vi "WS1050_Bench_Full Step_Hex_Characterization.vi"(4 "Send":bool, 5 "CLICK DOWN TO QUIT":bool=TRUE) -> (0 "EXE SEQ":bool, 1 "POWER ON":bool, 2 "CHARGE \nPUMP ON":bool, 3 "POWER OFF":bool)   [LabVIEW 2012]
panel:
  out "Con_HEX":string
  in  "Cmd Full":string[](array[string])=["01", "02", "03", "04", "05", "06", "07", "08", "09", "0A", "0B", "0C", "0D", "0E", "0F", "10", "11", "12", "13", "14", "15", "16", "17", "18", "19", "1A", "1B", "1C", "1D", "1E", "1F", "20", "21", "22", "23", "24", "25", "26", "27", "28", "29", "2A", "2B", "2C", "2D", "2E", "2F", "30", "31", "32", "33", "34", "35", "36", "37", "38", "39", "3A", "3B", "3A", "39", "38", "37", "36", "35", "34", "33", "32", "31", "30", "2F", "2E", "2D", "2C", "2B", "2A", "29", "28", "27", "26", "25", "24", "23", "22", "21", "20", "1F", "1E", "1D", "1C", "1B", "1A", "19", "18", "17", "16", "15", "14", "13", "12", "11", "10", "0F", "0E", "0D", "0C", "0B", "0A", "09", "08", "07", "06", "05", "04", "03", "02", "01", "00"]
  in  "Driver Name Full":string[](array[string])=["S0F1_UP", "S0F2_UP", "S0F12_UP", "S1_UP", "S1F1_UP", "S1F2_UP", "S1F12_UP", "S2_UP", "S2F1_UP", "S2F2_UP", "S2F12_UP", "S3_UP", "S3F1_UP", "S3F2_UP", "S3F12_UP", "S4_UP", "S4F1_UP", "S4F2_UP", "S4F12_UP", "S5_UP", "S5F1_UP", "S5F2_UP", "S5F12_UP", "S6_UP", "S6F1_UP", "S6F2_UP", "S6F12_UP", "S7_UP", "S7F1_UP", "S7F2_UP", "S7F12_UP", "S8_UP", "S8F1_UP", "S8F2_UP", "S8F12_UP", "S9_UP", "S9F1_UP", "S9F2_UP", "S9F12_UP", "S10_UP", "S10F1_UP", "S10F2_UP", "S10F12_UP", "S11_UP", "S11F1_UP", "S11F2_UP", "S11F12_UP", "S12_UP", "S12F1_UP", "S12F2_UP", "S12F12_UP", "S13_UP", "S13F1_UP", "S13F2_UP", "S13F12_UP", "S14_UP", "S14F1_UP", "S14F2_UP", "S14F12_UP", "S14F2_DN", "S14F1_DN", "S14_DN", "S13F12_DN", "S13F2_DN", "S13F1_DN", "S13_DN", "S12F12_DN", "S12F2_DN", "S12F1_DN", "S12_DN", "S11F12_DN", "S11F2_DN", "S11F1_DN", "S11_DN", "S10F12_DN", "S10F2_DN", "S10F1_DN", "S10_DN", "S9F12_DN", "S9F2_DN", "S9F1_DN", "S9_DN", "S8F12_DN", "S8F2_DN", "S8F1_DN", "S8_DN", "S7F12_DN", "S7F2_DN", "S7F1_DN", "S7_DN", "S6F12_DN", "S6F2_DN", "S6F1_DN", "S6_DN", "S5F12_DN", "S5F2_DN", "S5F1_DN", "S5_DN", "S4F12_DN", "S4F2_DN", "S4F1_DN", "S4_DN", "S3F12_DN", "S3F2_DN", "S3F1_DN", "S3_DN", "S2F12_DN", "S2F2_DN", "S2F1_DN", "S2_DN", "S1F12_DN", "S1F2_DN", "S1F1_DN", "S1_DN", "S0F12_DN", "S0F2_DN", "S0F1_DN", "ALL_OFF"]
  in  "Reg1_Bit Cntrl 2":string[](array[string])=["01", "02", "04", "08", "10", "20", "40", "80", "03", "06", "0C", "D8", "33", "66", "CC", "07", "0E", "1C", "38", "70", "E0", "0F", "1E", "3C", "78", "F0", "1F", "3E", "7C", "F8", "3F", "7E", "FC", "7F", "FE", "FD", "FB", "F7", "EF", "DF", "BF", "7F", "FC", "F9", "F3", "E7", "CF", "9F", "3F", "F8", "F1", "E3", "C7", "8F", "1F", "F0", "E1", "C3", "87", "0F", "E0", "C1", "83", "07", "C0", "81", "03", "AA", "55", "00"]
  out "CMin C3(pF)":dbl=-3.580591796875
  out "Delta_C3(pF)":dbl=11.179992796875
  out "CMin C2(pF)":dbl=-3.6213935546875
  out "Delta_C2(pF)":dbl=11.0864185546875
  out "Delta_C1(pF)":dbl=10.1718988828125
  out "CMin C1(pF)":dbl=-3.1732548828125005
  in  "Tab Control":enum32{"Control", "Indicator", "Error Out"}(tab)=enum."Error Out"
  in  "TMN DC\\CAP Data Log File Path":path=path "C:/Andy/WS1050"
  out "2K Cycles":bool
  out "Pass /Fail?":bool=TRUE
  in  "Title":string="WS1050_Bench_Full Steps_Hex Characterization"
  in  "Allowed (pF)":dbl=1.9898
  out "Difference":dbl=0.4481318359374997
  out "IDD_Stdby (uA)":string="13.613068E+0"
  in  "CAP Meas":refnum<visa-resource-name>="COM6"
  out "C2Cal (pF)":dbl=-4.841817382812501
  out "C1Cal (pF)":dbl=-4.2473720703125
  out "C3Cal (pF)":dbl=-4.793201171875
  in  "Bench #":string="1A"
  in  "Init AD7747":bool
  out "% Delta Cap":dbl=146.61383156779658 format="%#_5g"
  in  "VDD \nSet Up":dbl=3.3 format="%.2p"
  out "C2":dbl=1.2202167968750004
  out "C3":dbl=1.2128818359375
  out "C1":dbl=1.0745839843749998
  out "HS \nCheck":bool
  in  "Delay Cap Meas":u32=100
  in  "A364X_VDD":refnum<visa-resource-name>="GPIB0::6::INSTR"
  in  "Ke2000_IDD":refnum<visa-resource-name>="GPIB0::9::INSTR"
  out "Sequence":i32(listbox)=117
  out "IDD_ALLON (uA)":string="59.150183E+0"
  out "IDD_ALLOFF (uA)":string="59.926765E+0"
  in  "CP Setting":i32(ring) items=["CP OFF", "CP ON", "DVA OFF", "DVA ON", "ECAL OFF", "ECAL ON", "CP 40.25V", "CP 35V", "CP 38V", "CP 44V", "CP 50V", "CP 23.75V", "CP 25.25V", "CP 29.75V", "C1 ON", "C1 OFF", "C2 ON", "C2 OFF", "C3 ON", "C3 OFF"]
  out "Bins":string="111111111"
  in  "Calib\nSocket":bool
  in  "RFFE":refnum<visa-resource-name>="COM5"
  out "S_ValueC2(pF)":dbl=-4.841817382812501
  out "S_ValueC1(pF)":dbl=-4.2473720703125
  out "S_ValueC3(pF)":dbl=-4.793201171875
  out "Status":string="Idle....."
  in  "CMOS Setup":T1={"ECAL"=FALSE, "2K Cycles"=FALSE, "DVA"=FALSE, "EFuse RB"=TRUE, "Init RB"=TRUE, "HS Test"=FALSE}
  in  "Comment":string="Init Run"
  in  "Delta C Target":dbl=22.125
  in  "IDD Limit":dbl=0.02 format="%.2p"
  out "CMOS Out":T2={"ECAL"=FALSE, "DVA"=FALSE, "2K Cycles"=FALSE, "EFuse RB"=TRUE, "Init RB"=TRUE, "HS Test"=FALSE}
  out "Pass/Fail":bool
  in  "START \nTEST":bool
  in  "Idd Low (uA)":dbl
  in  "Idd High (uA)":dbl=3000.0
  in  "I Stby Limit (uA)":dbl=100.0
  in  "Header Table":string[][](table)=[["Lot#", "Wafer#", "SN#", "", "", "", "", "", "I_total"], ["WS1050", "T7", "1", "", "", "", "", "", "0.000000E+0"]]
  out "C1 Graph":dbl[](graph)=[0.0, 1.215518, 1.337774, 1.479006, 1.477455, 1.618706, 1.740946, 1.882279, 1.85507, 1.996156, 2.117995, 2.259391, 2.302419, 2.443647, 2.565752, 2.706903, 2.629912, 2.771129, 2.893216, 3.034232, 2.942072, 3.083374, 3.205229, 3.346353, 3.359243, 3.500349, 3.622406, 3.763442, 3.801931, 3.943032, 4.065077, 4.206051, 4.15953, 4.300568, 4.422481, 4.563321, 4.598434, 4.73931, 4.861127, 5.002075, 5.07149, 5.212336, 5.334259, 5.47494, 5.374126, 5.515039, 5.636803, 5.777399, 5.823291, 5.964162, 6.085894, 6.226579, 6.196894, 6.337836, 6.459297, 6.600081, 6.595847, 6.736394, 6.858027, 6.998644, 6.858178, 6.736639, 6.596258, 6.600357, 6.459984, 6.338313, 6.197737, 6.227304, 6.086547, 5.965041, 5.824373, 5.778321, 5.637963, 5.51618, 5.375233, 5.476038, 5.335547, 5.213573, 5.072775, 5.003335, 4.862609, 4.740632, 4.599788, 4.564702, 4.423796, 4.30184, 4.160986, 4.207129, 4.06623, 3.944312, 3.803315, 3.764714, 3.623703, 3.501688, 3.360495, 3.34748, 3.206586, 3.08447, 2.94347, 3.035012, 2.893932, 2.771681, 2.630812, 2.707732, 2.566481, 2.444467, 2.303202, 2.259867, 2.118534, 1.996384, 1.855069, 1.882756, 1.741472, 1.619091, 1.477851, 1.479718, 1.338271, 1.216057, 1.074723]
  out "C3 Graph":dbl[](graph)=[0.0, 1.361336, 1.484217, 1.6328, 1.621303, 1.769957, 1.892482, 2.041041, 1.989155, 2.137771, 2.260655, 2.409242, 2.44755, 2.595912, 2.718779, 2.867148, 2.818958, 2.967286, 3.089997, 3.238399, 3.289025, 3.437506, 3.560199, 3.708618, 3.662552, 3.81095, 3.934051, 4.082135, 4.106606, 4.254703, 4.377176, 4.525365, 4.541886, 4.690311, 4.812674, 4.960813, 4.989934, 5.13817, 5.260637, 5.40866, 5.476124, 5.624491, 5.746858, 5.89501, 5.889363, 6.037764, 6.160056, 6.30779, 6.334885, 6.482729, 6.604835, 6.752733, 6.698209, 6.84634, 6.968445, 7.11599, 7.181717, 7.329828, 7.45165, 7.599401, 7.452068, 7.330011, 7.182202, 7.11678, 6.968958, 6.846465, 6.698591, 6.753367, 6.605286, 6.482884, 6.335051, 6.308537, 6.16111, 6.038187, 5.890584, 5.895679, 5.747959, 5.625363, 5.477302, 5.409548, 5.2619, 5.139239, 4.991471, 4.961949, 4.813866, 4.691039, 4.542875, 4.526602, 4.378426, 4.255908, 4.10765, 4.083617, 3.935409, 3.812553, 3.664153, 3.709927, 3.561527, 3.438792, 3.290498, 3.240085, 3.091945, 2.968868, 2.820536, 2.869053, 2.720493, 2.59781, 2.44922, 2.410599, 2.262307, 2.13926, 1.990714, 2.042517, 1.894032, 1.770843, 1.622592, 1.633918, 1.485479, 1.362411, 1.21368]
  out "C2 Graph":dbl[](graph)=[0.0, 1.364697, 1.516186, 1.660924, 1.655455, 1.800099, 1.951666, 2.096205, 2.009943, 2.154575, 2.306069, 2.450681, 2.492821, 2.637354, 2.788981, 2.933582, 2.920825, 3.065458, 3.217283, 3.361717, 3.352427, 3.49727, 3.648553, 3.792817, 3.814088, 3.958804, 4.110113, 4.25463, 4.067543, 4.212351, 4.364132, 4.508611, 4.394954, 4.539699, 4.6909, 4.835606, 4.861541, 5.006121, 5.157679, 5.302112, 5.288999, 5.434083, 5.585449, 5.730307, 5.699932, 5.844717, 5.995834, 6.140104, 6.170777, 6.315693, 6.466977, 6.611707, 6.553808, 6.698186, 6.849589, 6.994114, 7.023831, 7.168418, 7.320228, 7.465025, 7.320119, 7.168711, 7.024116, 6.994523, 6.850515, 6.699219, 6.554088, 6.612322, 6.467537, 6.316291, 6.17185, 6.141468, 5.997138, 5.845646, 5.70093, 5.730797, 5.586201, 5.435164, 5.290619, 5.303903, 5.158995, 5.007956, 4.862967, 4.837034, 4.692302, 4.54089, 4.396507, 4.509821, 4.365486, 4.214033, 4.069551, 4.255679, 4.11138, 3.960171, 3.81544, 3.794067, 3.649285, 3.498325, 3.353707, 3.362646, 3.21808, 3.066712, 2.922035, 2.934946, 2.790031, 2.638727, 2.493927, 2.451741, 2.307302, 2.156018, 2.011369, 2.097184, 1.952486, 1.801188, 1.656408, 1.662095, 1.517303, 1.365852, 1.221114]
  out "Init EFuse RB":string[](array[string])=["00", "00", "00", "00", "00", "00", "00", "00", "00", "00"]
  out "EFuse 1":string="00"
  out "EFuse 2":string="00"
  out "I_stdby End":string="29.576433E+0"
  out "RB All Regs Dump":string[](array[string])=["00", "00", "00", "00", "00", "00", "00", "00", "00", "00", "00", "00", "00", "00", "00", "00", "00", "00", "00", "00"]
  in  "RB All Regs":bool=TRUE
  out "HEX":string="4811EA"
  out "RFFE Out":errorcluster={"status"=FALSE, "code"=1073676418, "source"="VISA Close in WS1050_Bench_Full Step_Hex_Characterization.vi"}
  out "I2C Error Out":errorcluster={"status"=FALSE, "code"=1073676294, "source"="VISA Read in PIC_Write_Read _AD7747.vi->WS1050_AD7747_MeasCAP_Ver1.1.vi->WS1050_AD7747_Control_Cap_bank_Measure Ver1.0.vi->WS1050_Bench_Full Step_Hex_Characterization.vi"}
  out "After 2K Cycles":errorcluster={"status"=FALSE, "code"=1073676294, "source"="VISA Read in PIC_Write_Read _AD7747.vi->WS1050_AD7747_MeasCAP_Ver1.1.vi->WS1050_AD7747_Control_Cap_bank_Measure Ver1.0.vi->WS1050_Bench_Full Step_Hex_Characterization.vi"}
  out "B4 While Loop":errorcluster
  out "B4 Init RB":errorcluster={"status"=FALSE, "code"=1073676294, "source"="VISA Read in PIC_Write_Read _AD7747.vi->WS1050_AD7747_MeasCAP_Ver1.1.vi->WS1050_AD7747_Control_Cap_bank_Measure Ver1.0.vi->WS1050_Bench_Full Step_Hex_Characterization.vi"}
  out "After EFuse RB":errorcluster={"status"=FALSE, "code"=1073676294, "source"="VISA Read in PIC_Write_Read _AD7747.vi->WS1050_AD7747_MeasCAP_Ver1.1.vi->WS1050_AD7747_Control_Cap_bank_Measure Ver1.0.vi->WS1050_Bench_Full Step_Hex_Characterization.vi"}
  out "Power OFF":errorcluster={"status"=FALSE, "code"=1073676294, "source"="VISA Read in PIC_Write_Read _AD7747.vi->WS1050_AD7747_MeasCAP_Ver1.1.vi->WS1050_AD7747_Control_Cap_bank_Measure Ver1.0.vi->WS1050_Bench_Full Step_Hex_Characterization.vi"}
  out "After C1":errorcluster={"status"=FALSE, "code"=1073676294, "source"="VISA Read in PIC_Write_Read _AD7747.vi->AD7747_Meas_HEXCAP.vi->WS1050_Bench_Full Step_Hex_Characterization.vi"}
  out "After C2":errorcluster={"status"=FALSE, "code"=1073676294, "source"="VISA Read in PIC_Write_Read _AD7747.vi->AD7747_Meas_HEXCAP.vi->WS1050_Bench_Full Step_Hex_Characterization.vi"}
  out "Ater C3":errorcluster={"status"=FALSE, "code"=1073676294, "source"="VISA Read in PIC_Write_Read _AD7747.vi->AD7747_Meas_HEXCAP.vi->WS1050_Bench_Full Step_Hex_Characterization.vi"}
  out "VDD Out Dup":refnum<visa-resource-name>="GPIB0::6::INSTR"
  out "After Cmin":errorcluster={"status"=FALSE, "code"=1073676294, "source"="VISA Read in PIC_Write_Read _AD7747.vi->AD7747_Meas_HEXCAP.vi->WS1050_Bench_Full Step_Hex_Characterization.vi"}
  out "Completed":errorcluster={"status"=FALSE, "code"=1073676294, "source"="VISA Read in PIC_Write_Read _AD7747.vi->AD7747_Meas_HEXCAP.vi->WS1050_Bench_Full Step_Hex_Characterization.vi"}
  out "P/S Out":errorcluster={"status"=FALSE, "code"=1073676294, "source"="VISA Read in PIC_Write_Read _AD7747.vi->WS1050_AD7747_MeasCAP_Ver1.1.vi->WS1050_AD7747_Control_Cap_bank_Measure Ver1.0.vi->WS1050_Bench_Full Step_Hex_Characterization.vi"}
  out "RFFE Out After Test":errorcluster={"status"=FALSE, "code"=1073676294, "source"="VISA Read in PIC_Write_Read _AD7747.vi->AD7747_Meas_HEXCAP.vi->WS1050_Bench_Full Step_Hex_Characterization.vi"}
  out "All Out":string[](array[string])=["4/6/2015", "2:30:56 PM", "WS1050", "T7", "1", "00", "00", "00", "00", "00", "00", "00", "00", "00", "00", "OFF", "00", "00", "13.613068E+0", "59.150183E+0", "59.926765E+0", "1.074117E+0", "1.220424E+0", "1.212609E+0", "1.215518E+0", "50A095", "1.337774E+0", "52899C", "1.479006E+0", "54BE89", "1.477455E+0", "54B855", "1.618706E+0", "56ED56", "1.740946E+0", "58D64C", "1.882279E+0", "5B0BA1", "1.855070E+0", "5A9ECB", "1.996156E+0", "5CD323", "2.117995E+0", "5EBA7E", "2.259391E+0", "60F013", "2.302419E+0", "619C30", "2.443647E+0", "63D11A", "2.565752E+0", "65B985", "2.706903E+0", "67EE20", "2.629912E+0", "66BA29", "2.771129E+0", "68EF07", "2.893216E+0", "6AD760", "3.034232E+0", "6D0B71", "2.942072E+0", "6B9ACD", "3.083374E+0", "6DD002", "3.205229E+0", "6FB76E", "3.346353E+0", "71EBEC", "3.359243E+0", "721F7C", "3.500349E+0", "7453E8", "3.622406E+0", "763C23", "3.763442E+0", "787048", "3.801931E+0", "790A3C", "3.943032E+0", "7B3EA4", "4.065077E+0", "7D26D2", "4.206051E+0", "7F5AB7", "4.159530E+0", "7EA0A2", "4.300568E+0", "80D4C9", "4.422481E+0", "82BC70", "4.563321E+0", "84EFCC", "4.598434E+0", "857C3F", "4.739310E+0", "87AFC0", "4.861127E+0", "899705", "5.002075E+0", "8BCAD0", "5.071490E+0", "8CE079", "5.212336E+0", "8F13DB", "5.334259E+0", "90FB8C", "5.474940E+0", "932E46", "5.374126E+0", "919B04", "5.515039E+0", "93CEAB", "5.636803E+0", "95B5B9", "5.777399E+0", "97E81C", "5.823291E+0", "989FAD", "5.964162E+0", "9AD329", "6.085894E+0", "9CBA16", "6.226579E+0", "9EECD4", "6.196894E+0", "9E7616", "6.337836E+0", "A0A9DB", "6.459297E+0", "A28FB3", "6.600081E+0", "A4C2D6", "6.595847E+0", "A4B1E6", "6.736394E+0", "A6E416", "6.858027E+0", "A8CA9F", "6.998644E+0", "AAFD16", "6.858178E+0", "A8CB39", "6.736639E+0", "A6E511", "6.596258E+0", "A4B38B", "6.600357E+0", "A4C3F1", "6.459984E+0", "A29273", "6.338313E+0", "A0ABC4", "6.197737E+0", "9E7976", "6.227304E+0", "9EEFBA", "6.086547E+0", "9CBCB3", "5.965041E+0", "9AD6AD", "5.824373E+0", "98A401", "5.778321E+0", "97EBCC", "5.637963E+0", "95BA5D", "5.516180E+0", "93D33B", "5.375233E+0", "919F72", "5.476038E+0", "9332AA", "5.335547E+0", "9100B3", "5.213573E+0", "8F18CE", "5.072775E+0", "8CE59D", "5.003335E+0", "8BCFDA", "4.862609E+0", "899CF3", "4.740632E+0", "87B50A", "4.599788E+0", "8581AA", "4.564702E+0", "84F552", "4.423796E+0", "82C1B2", "4.301840E+0", "80D9DF", "4.160986E+0", "7EA675", "4.207129E+0", "7F5F07", "4.066230E+0", "7D2B6F", "3.944312E+0", "7B43C2", "3.803315E+0", "790FC6", "3.764714E+0", "78755E", "3.623703E+0", "764153", "3.501688E+0", "745944", "3.360495E+0", "72247E", "3.347480E+0", "71F06F", "3.206586E+0", "6FBCDB", "3.084470E+0", "6DD464", "2.943470E+0", "6BA064", "3.035012E+0", "6D0E8F", "2.893932E+0", "6ADA3D", "2.771681E+0", "68F13C", "2.630812E+0", "66BDC2", "2.707732E+0", "67F171", "2.566481E+0", "65BC70", "2.444467E+0", "63D461", "2.303202E+0", "619F52", "2.259867E+0", "60F1FB", "2.118534E+0", "5EBCA6", "1.996384E+0", "5CD40C", "1.855069E+0", "5A9ECA", "1.882756E+0", "5B0D89", "1.741472E+0", "58D866", "1.619091E+0", "56EEE0", "1.477851E+0", "54B9EA", "1.479718E+0", "54C162", "1.338271E+0", "528B98", "1.216057E+0", "50A2BD", "1.074723E+0", "4E6D67", "4.388773E+0", "4.511029E+0", "4.652261E+0", "4.650710E+0", "4.791961E+0", "4.914201E+0", "5.055534E+0", "5.028325E+0", "5.169411E+0", "5.291250E+0", "5.432646E+0", "5.475674E+0", "5.616902E+0", "5.739007E+0", "5.880158E+0", "5.803167E+0", "5.944384E+0", "6.066471E+0", "6.207487E+0", "6.115327E+0", "6.256629E+0", "6.378484E+0", "6.519608E+0", "6.532498E+0", "6.673604E+0", "6.795661E+0", "6.936697E+0", "6.975186E+0", "7.116287E+0", "7.238332E+0", "7.379306E+0", "7.332785E+0", "7.473823E+0", "7.595736E+0", "7.736576E+0", "7.771689E+0", "7.912565E+0", "8.034382E+0", "8.175330E+0", "8.244745E+0", "8.385591E+0", "8.507514E+0", "8.648195E+0", "8.547381E+0", "8.688294E+0", "8.810058E+0", "8.950654E+0", "8.996546E+0", "9.137417E+0", "9.259149E+0", "9.399834E+0", "9.370149E+0", "9.511091E+0", "9.632552E+0", "9.773336E+0", "9.769102E+0", "9.909649E+0", "1.003128E+1", "5.390000E-4", "4.970000E-4", "7.120000E-4", "3.960000E-4", "3.850000E-4", "5.260000E-4", "4.770000E-4", "-1.000000E-6", "2.280000E-4", "5.390000E-4", "4.760000E-4", "7.830000E-4", "8.200000E-4", "7.290000E-4", "8.290000E-4", "9.000000E-4", "5.520000E-4", "7.160000E-4", "7.800000E-4", "1.398000E-3", "1.096000E-3", "1.357000E-3", "1.127000E-3", "1.252000E-3", "1.339000E-3", "1.297000E-3", "1.272000E-3", "1.384000E-3", "1.280000E-3", "1.153000E-3", "1.078000E-3", "1.456000E-3", "1.272000E-3", "1.315000E-3", "1.381000E-3", "1.354000E-3", "1.322000E-3", "1.482000E-3", "1.260000E-3", "1.285000E-3", "1.237000E-3", "1.288000E-3", "1.098000E-3", "1.107000E-3", "1.141000E-3", "1.160000E-3", "9.220000E-4", "1.082000E-3", "8.790000E-4", "6.530000E-4", "7.250000E-4", "8.430000E-4", "4.770000E-4", "6.870000E-4", "2.760000E-4", "4.110000E-4", "2.450000E-4", "1.510000E-4", "1.364697E+0", "49AB85", "1.516186E+0", "4C0979", "1.660924E+0", "4E4C6D", "1.655455E+0", "4E368D", "1.800099E+0", "507920", "1.951666E+0", "52D765", "2.096205E+0", "55198D", "2.009943E+0", "53C081", "2.154575E+0", "560308", "2.306069E+0", "586102", "2.450681E+0", "5AA374", "2.492821E+0", "5B4C04", "2.637354E+0", "5D8E26", "2.788981E+0", "5FECA8", "2.933582E+0", "622F0F", "2.920825E+0", "61FC08", "3.065458E+0", "643E90", "3.217283E+0", "669DDD", "3.361717E+0", "68DF99", "3.352427E+0", "68BA70", "3.497270E+0", "6AFDCF", "3.648553E+0", "6D5AF1", "3.792817E+0", "6F9C00", "3.814088E+0", "6FF115", "3.958804E+0", "7233F2", "4.110113E+0", "74912F", "4.254630E+0", "76D340", "4.067543E+0", "73E6E7", "4.212351E+0", "762A22", "4.364132E+0", "788942", "4.508611E+0", "7ACB2D", "4.394954E+0", "79048C", "4.539699E+0", "7B4787", "4.690900E+0", "7DA455", "4.835606E+0", "7FE728", "4.861541E+0", "804EE5", "5.006121E+0", "829137", "5.157679E+0", "84EF72", "5.302112E+0", "87312E", "5.288999E+0", "86FCBA", "5.434083E+0", "894110", "5.585449E+0", "8B9E87", "5.730307E+0", "8DE1F5", "5.699932E+0", "8D6875", "5.844717E+0", "8FAB99", "5.995834E+0", "920811", "6.140104E+0", "944925", "6.170777E+0", "94C3D7", "6.315693E+0", "970781", "6.466977E+0", "9964A3", "6.611707E+0", "9BA78F", "6.553808E+0", "9ABFF6", "6.698186E+0", "9D0179", "6.849589E+0", "9F5F16", "6.994114E+0", "A1A130", "7.023831E+0", "A2180E", "7.168418E+0", "A45A67", "7.320228E+0", "A6B9A4", "7.465025E+0", "A8FCD5", "7.320119E+0", "A6B935", "7.168711E+0", "A45B93", "7.024116E+0", "A21932", "6.994523E+0", "A1A2D3", "6.850515E+0", "9F62CA", "6.699219E+0", "9D059B", "6.554088E+0", "9AC115", "6.612322E+0", "9BAA05", "6.467537E+0", "9966E1", "6.316291E+0", "9709E5", "6.171850E+0", "94C821", "6.141468E+0", "944E9A", "5.997138E+0", "920D48", "5.845646E+0", "8FAF50", "5.700930E+0", "8D6C73", "5.730797E+0", "8DE3EB", "5.586201E+0", "8BA189", "5.435164E+0", "894563", "5.290619E+0", "870335", "5.303903E+0", "873858", "5.158995E+0", "84F4B6", "5.007956E+0", "82988E", "4.862967E+0", "805499", "4.837034E+0", "7FECDE", "4.692302E+0", "7DA9F0", "4.540890E+0", "7B4C4A", "4.396507E+0", "790AC2", "4.509821E+0", "7AD004", "4.365486E+0", "788EAD", "4.214033E+0", "7630DD", "4.069551E+0", "73EEEF", "4.255679E+0", "76D772", "4.111380E+0", "749640", "3.960171E+0", "72396A", "3.815440E+0", "6FF67E", "3.794067E+0", "6FA100", "3.649285E+0", "6D5DDF", "3.498325E+0", "6B0208", "3.353707E+0", "68BF8F", "3.362646E+0", "68E350", "3.218080E+0", "66A10D", "3.066712E+0", "644394", "2.922035E+0", "6200DF", "2.934946E+0", "623484", "2.790031E+0", "5FF0DB", "2.638727E+0", "5D93A3", "2.493927E+0", "5B5070", "2.451741E+0", "5AA7B2", "2.307302E+0", "5865F0", "2.156018E+0", "5608CD", "2.011369E+0", "53C635", "2.097184E+0", "551D77", "1.952486E+0", "52DAAD", "1.801188E+0", "507D7B", "1.656408E+0", "4E3A5D", "1.662095E+0", "4E511C", "1.517303E+0", "4C0DF1", "1.365852E+0", "49B023", "1.221114E+0", "476D30", "4.986091E+0", "5.137580E+0", "5.282318E+0", "5.276849E+0", "5.421493E+0", "5.573060E+0", "5.717599E+0", "5.631337E+0", "5.775969E+0", "5.927463E+0", "6.072075E+0", "6.114215E+0", "6.258748E+0", "6.410375E+0", "6.554976E+0", "6.542219E+0", "6.686852E+0", "6.838677E+0", "6.983111E+0", "6.973821E+0", "7.118664E+0", "7.269947E+0", "7.414211E+0", "7.435482E+0", "7.580198E+0", "7.731507E+0", "7.876024E+0", "7.688937E+0", "7.833745E+0", "7.985526E+0", "8.130005E+0", "8.016348E+0", "8.161093E+0", "8.312294E+0", "8.457000E+0", "8.482935E+0", "8.627515E+0", "8.779073E+0", "8.923506E+0", "8.910393E+0", "9.055477E+0", "9.206843E+0", "9.351701E+0", "9.321326E+0", "9.466111E+0", "9.617228E+0", "9.761498E+0", "9.792171E+0", "9.937087E+0", "1.008837E+1", "1.023310E+1", "1.017520E+1", "1.031958E+1", "1.047098E+1", "1.061551E+1", "1.064522E+1", "1.078981E+1", "1.094162E+1", "1.155000E-3", "1.117000E-3", "1.171000E-3", "9.530000E-4", "1.089000E-3", "8.200000E-4", "9.790000E-4", "1.426000E-3", "1.443000E-3", "1.233000E-3", "1.060000E-3", "1.106000E-3", "1.373000E-3", "1.050000E-3", "1.364000E-3", "1.210000E-3", "1.254000E-3", "7.970000E-4", "9.290000E-4", "1.280000E-3", "1.055000E-3", "7.320000E-4", "1.250000E-3", "1.352000E-3", "1.367000E-3", "1.267000E-3", "1.049000E-3", "2.008000E-3", "1.682000E-3", "1.354000E-3", "1.210000E-3", "1.553000E-3", "1.191000E-3", "1.402000E-3", "1.428000E-3", "1.426000E-3", "1.835000E-3", "1.316000E-3", "1.791000E-3", "1.620000E-3", "1.081000E-3", "7.520000E-4", "4.900000E-4", "9.980000E-4", "9.290000E-4", "1.304000E-3", "1.364000E-3", "1.073000E-3", "5.980000E-4", "5.600000E-4", "6.150000E-4", "2.800000E-4", "1.033000E-3", "9.260000E-4", "4.090000E-4", "2.850000E-4", "2.930000E-4", "-1.090000E-4", "1.361336E+0", "4A608A", "1.484217E+0", "4C4C10", "1.632800E+0", "4E9E65", "1.621303E+0", "4E7068", "1.769957E+0", "50C306", "1.892482E+0", "52AD20", "2.041041E+0", "54FF5C", "1.989155E+0", "542FD1", "2.137771E+0", "568247", "2.260655E+0", "586DD1", "2.409242E+0", "5AC02A", "2.447550E+0", "5B5965", "2.595912E+0", "5DAAD8", "2.718779E+0", "5F9650", "2.867148E+0", "61E7CA", "2.818958E+0", "612707", "2.967286E+0", "637857", "3.089997E+0", "65632F", "3.238399E+0", "67B4CB", "3.289025E+0", "687F4C", "3.437506E+0", "6AD138", "3.560199E+0", "6CBBFE", "3.708618E+0", "6F0DAB", "3.662552E+0", "6E5567", "3.810950E+0", "70A6FF", "3.934051E+0", "729366", "4.082135E+0", "74E3BC", "4.106606E+0", "75459F", "4.254703E+0", "779602", "4.377176E+0", "797FE6", "4.525365E+0", "7BD0A8", "4.541886E+0", "7C12BD", "4.690311E+0", "7E6470", "4.812674E+0", "804DE4", "4.960813E+0", "829E73", "4.989934E+0", "8312EE", "5.138170E+0", "8563E0", "5.260637E+0", "874DBE", "5.408660E+0", "899DD6", "5.476124E+0", "8AABB1", "5.624491E+0", "8CFD29", "5.746858E+0", "8EE6A1", "5.895010E+0", "91373C", "5.889363E+0", "9120A6", "6.037764E+0", "937240", "6.160056E+0", "955B6B", "6.307790E+0", "97AA5B", "6.334885E+0", "9816BC", "6.482729E+0", "9A661C", "6.604835E+0", "9C4E89", "6.752733E+0", "9E9E21", "6.698209E+0", "9DC408", "6.846340E+0", "A0148E", "6.968445E+0", "A1FCFA", "7.115990E+0", "A44B28", "7.181717E+0", "A55210", "7.329828E+0", "A7A282", "7.451650E+0", "A989CC", "7.599401E+0", "ABD8CD", "7.452068E+0", "A98B78", "7.330011E+0", "A7A33D", "7.182202E+0", "A55401", "7.116780E+0", "A44E51", "6.968958E+0", "A1FF07", "6.846465E+0", "A0150E", "6.698591E+0", "9DC58F", "6.753367E+0", "9EA0AA", "6.605286E+0", "9C5057", "6.482884E+0", "9A66BB", "6.335051E+0", "981766", "6.308537E+0", "97AD58", "6.161110E+0", "955FA3", "6.038187E+0", "9373F1", "5.890584E+0", "912588", "5.895679E+0", "9139E9", "5.747959E+0", "8EEB08", "5.625363E+0", "8D00A6", "5.477302E+0", "8AB067", "5.409548E+0", "89A163", "5.261900E+0", "8752CC", "5.139239E+0", "856827", "4.991471E+0", "831914", "4.961949E+0", "82A2FE", "4.813866E+0", "8052A9", "4.691039E+0", "7E675A", "4.542875E+0", "7C16B2", "4.526602E+0", "7BD59A", "4.378426E+0", "7984E6", "4.255908E+0", "779AD4", "4.107650E+0", "7549CC", "4.083617E+0", "74E9AA", "3.935409E+0", "7298D5", "3.812553E+0", "70AD68", "3.664153E+0", "6E5BCF", "3.709927E+0", "6F12E7", "3.561527E+0", "6CC14E", "3.438792E+0", "6AD65D", "3.290498E+0", "688530", "3.240085E+0", "67BB89", "3.091945E+0", "656AFA", "2.968868E+0", "637EAB", "2.820536E+0", "612D57", "2.869053E+0", "61EF68", "2.720493E+0", "5F9D2B", "2.597810E+0", "5DB26F", "2.449220E+0", "5B6013", "2.410599E+0", "5AC597", "2.262307E+0", "58746C", "2.139260E+0", "56883C", "1.990714E+0", "54360D", "2.042517E+0", "550543", "1.894032E+0", "52B353", "1.770843E+0", "50C691", "1.622592E+0", "4E7590", "1.633918E+0", "4EA2DE", "1.485479E+0", "4C511C", "1.362411E+0", "4A64D7", "1.213680E+0", "4811EA", "4.941928E+0", "5.064809E+0", "5.213392E+0", "5.201895E+0", "5.350549E+0", "5.473074E+0", "5.621633E+0", "5.569747E+0", "5.718363E+0", "5.841247E+0", "5.989834E+0", "6.028142E+0", "6.176504E+0", "6.299371E+0", "6.447740E+0", "6.399550E+0", "6.547878E+0", "6.670589E+0", "6.818991E+0", "6.869617E+0", "7.018098E+0", "7.140791E+0", "7.289210E+0", "7.243144E+0", "7.391542E+0", "7.514643E+0", "7.662727E+0", "7.687198E+0", "7.835295E+0", "7.957768E+0", "8.105957E+0", "8.122478E+0", "8.270903E+0", "8.393266E+0", "8.541405E+0", "8.570526E+0", "8.718762E+0", "8.841229E+0", "8.989252E+0", "9.056716E+0", "9.205083E+0", "9.327450E+0", "9.475602E+0", "9.469955E+0", "9.618356E+0", "9.740648E+0", "9.888382E+0", "9.915477E+0", "1.006332E+1", "1.018543E+1", "1.033332E+1", "1.027880E+1", "1.042693E+1", "1.054904E+1", "1.069658E+1", "1.076231E+1", "1.091042E+1", "1.103224E+1", "1.075000E-3", "1.262000E-3", "1.118000E-3", "1.289000E-3", "8.860000E-4", "1.550000E-3", "1.476000E-3", "1.559000E-3", "1.489000E-3", "1.652000E-3", "1.357000E-3", "1.670000E-3", "1.898000E-3", "1.714000E-3", "1.905000E-3", "1.578000E-3", "1.582000E-3", "1.948000E-3", "1.686000E-3", "1.473000E-3", "1.286000E-3", "1.328000E-3", "1.309000E-3", "1.601000E-3", "1.603000E-3", "1.358000E-3", "1.482000E-3", "1.044000E-3", "1.205000E-3", "1.250000E-3", "1.237000E-3", "9.890000E-4", "7.280000E-4", "1.192000E-3", "1.136000E-3", "1.537000E-3", "1.069000E-3", "1.263000E-3", "8.880000E-4", "1.178000E-3", "8.720000E-4", "1.101000E-3", "6.690000E-4", "1.221000E-3", "4.230000E-4", "1.054000E-3", "7.470000E-4", "1.660000E-4", "1.550000E-4", "4.510000E-4", "6.340000E-4", "3.820000E-4", "1.250000E-4", "5.130000E-4", "7.900000E-4", "4.850000E-4", "1.830000E-4", "4.180000E-4"]
  out "2K Out":errorcluster={"status"=FALSE, "code"=1073676418, "source"="VISA Close in WS1050_Bench_Full Step_Hex_Characterization.vi"}
  out "Lot":string="WS1050"
  out "Wafer":string="T7"
  out "C3(pF)":dbl=-8.192 format="%#_4g"
  out "C1(pF)":dbl=-8.192 format="%#_4g"
  out "C2(pF)":dbl=-8.192 format="%#_4g"
  in  "error in":errorcluster
  # "Company:  WiSpry Inc\n198 Fairbanks Ste 198 Irvine\n\nCreated by:  Andy V Tran\nDate:  04/02/2015\nTest Program:  WS1050 Bench\nFull Steps_Characterization\nLabVIEW 2012 Professional"
  # "Firmware:  Marketing V1.9\nTest Program :  WS1050_Bench_Full Step_Hex Characterization\nVSA: No\nVPI: No"
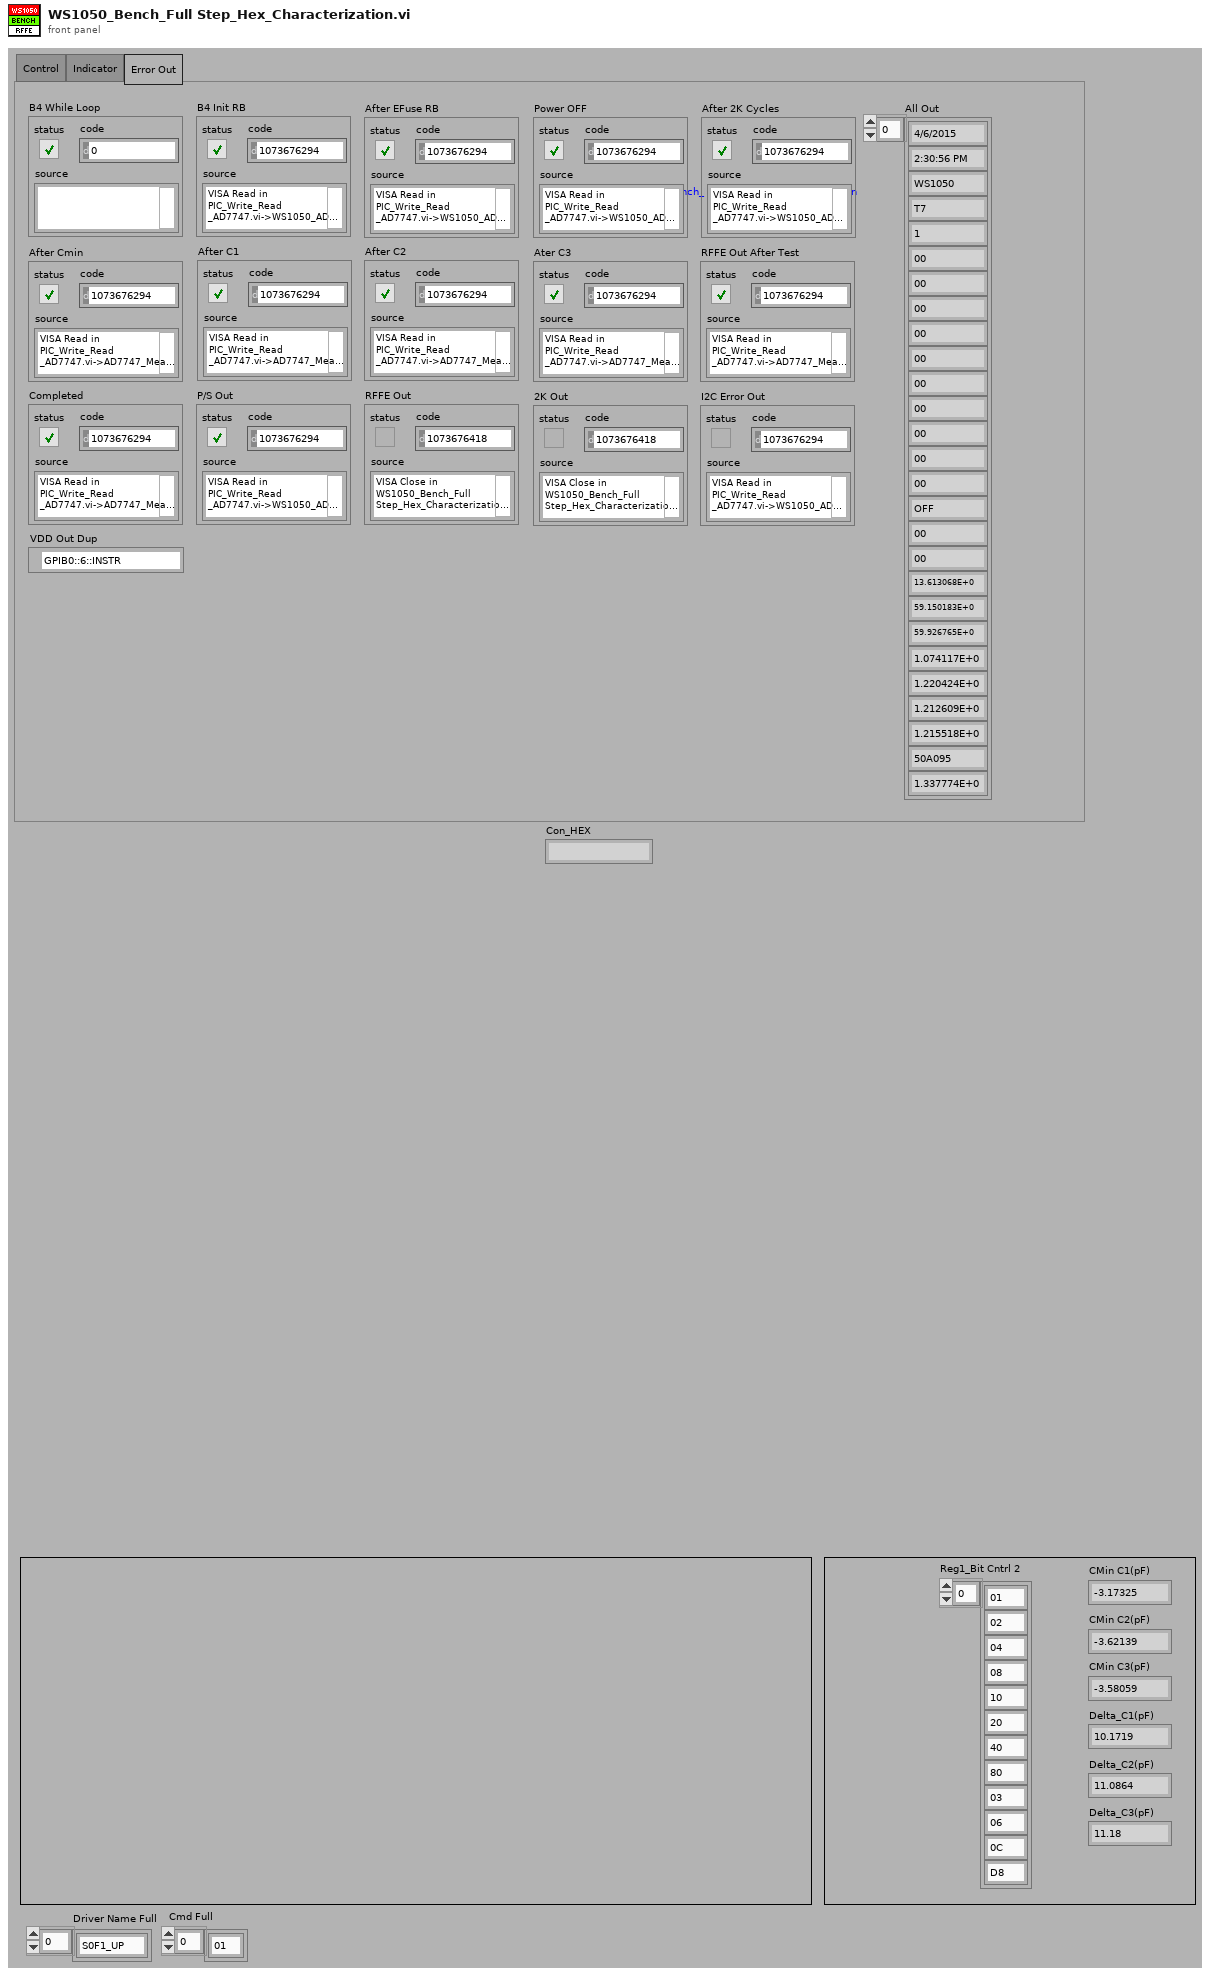
[diagram p1: front panel]
types:
  T1 = cluster{"ECAL":bool, "2K Cycles":bool, "DVA":bool, "EFuse RB":bool, "Init RB":bool, "HS Test":bool}
  T2 = cluster{"ECAL":bool, "DVA":bool, "2K Cycles":bool, "EFuse RB":bool, "Init RB":bool, "HS Test":bool}
  T3 = cluster{"Bench #":string, "Title ":string, "string":string, "Comment":string}
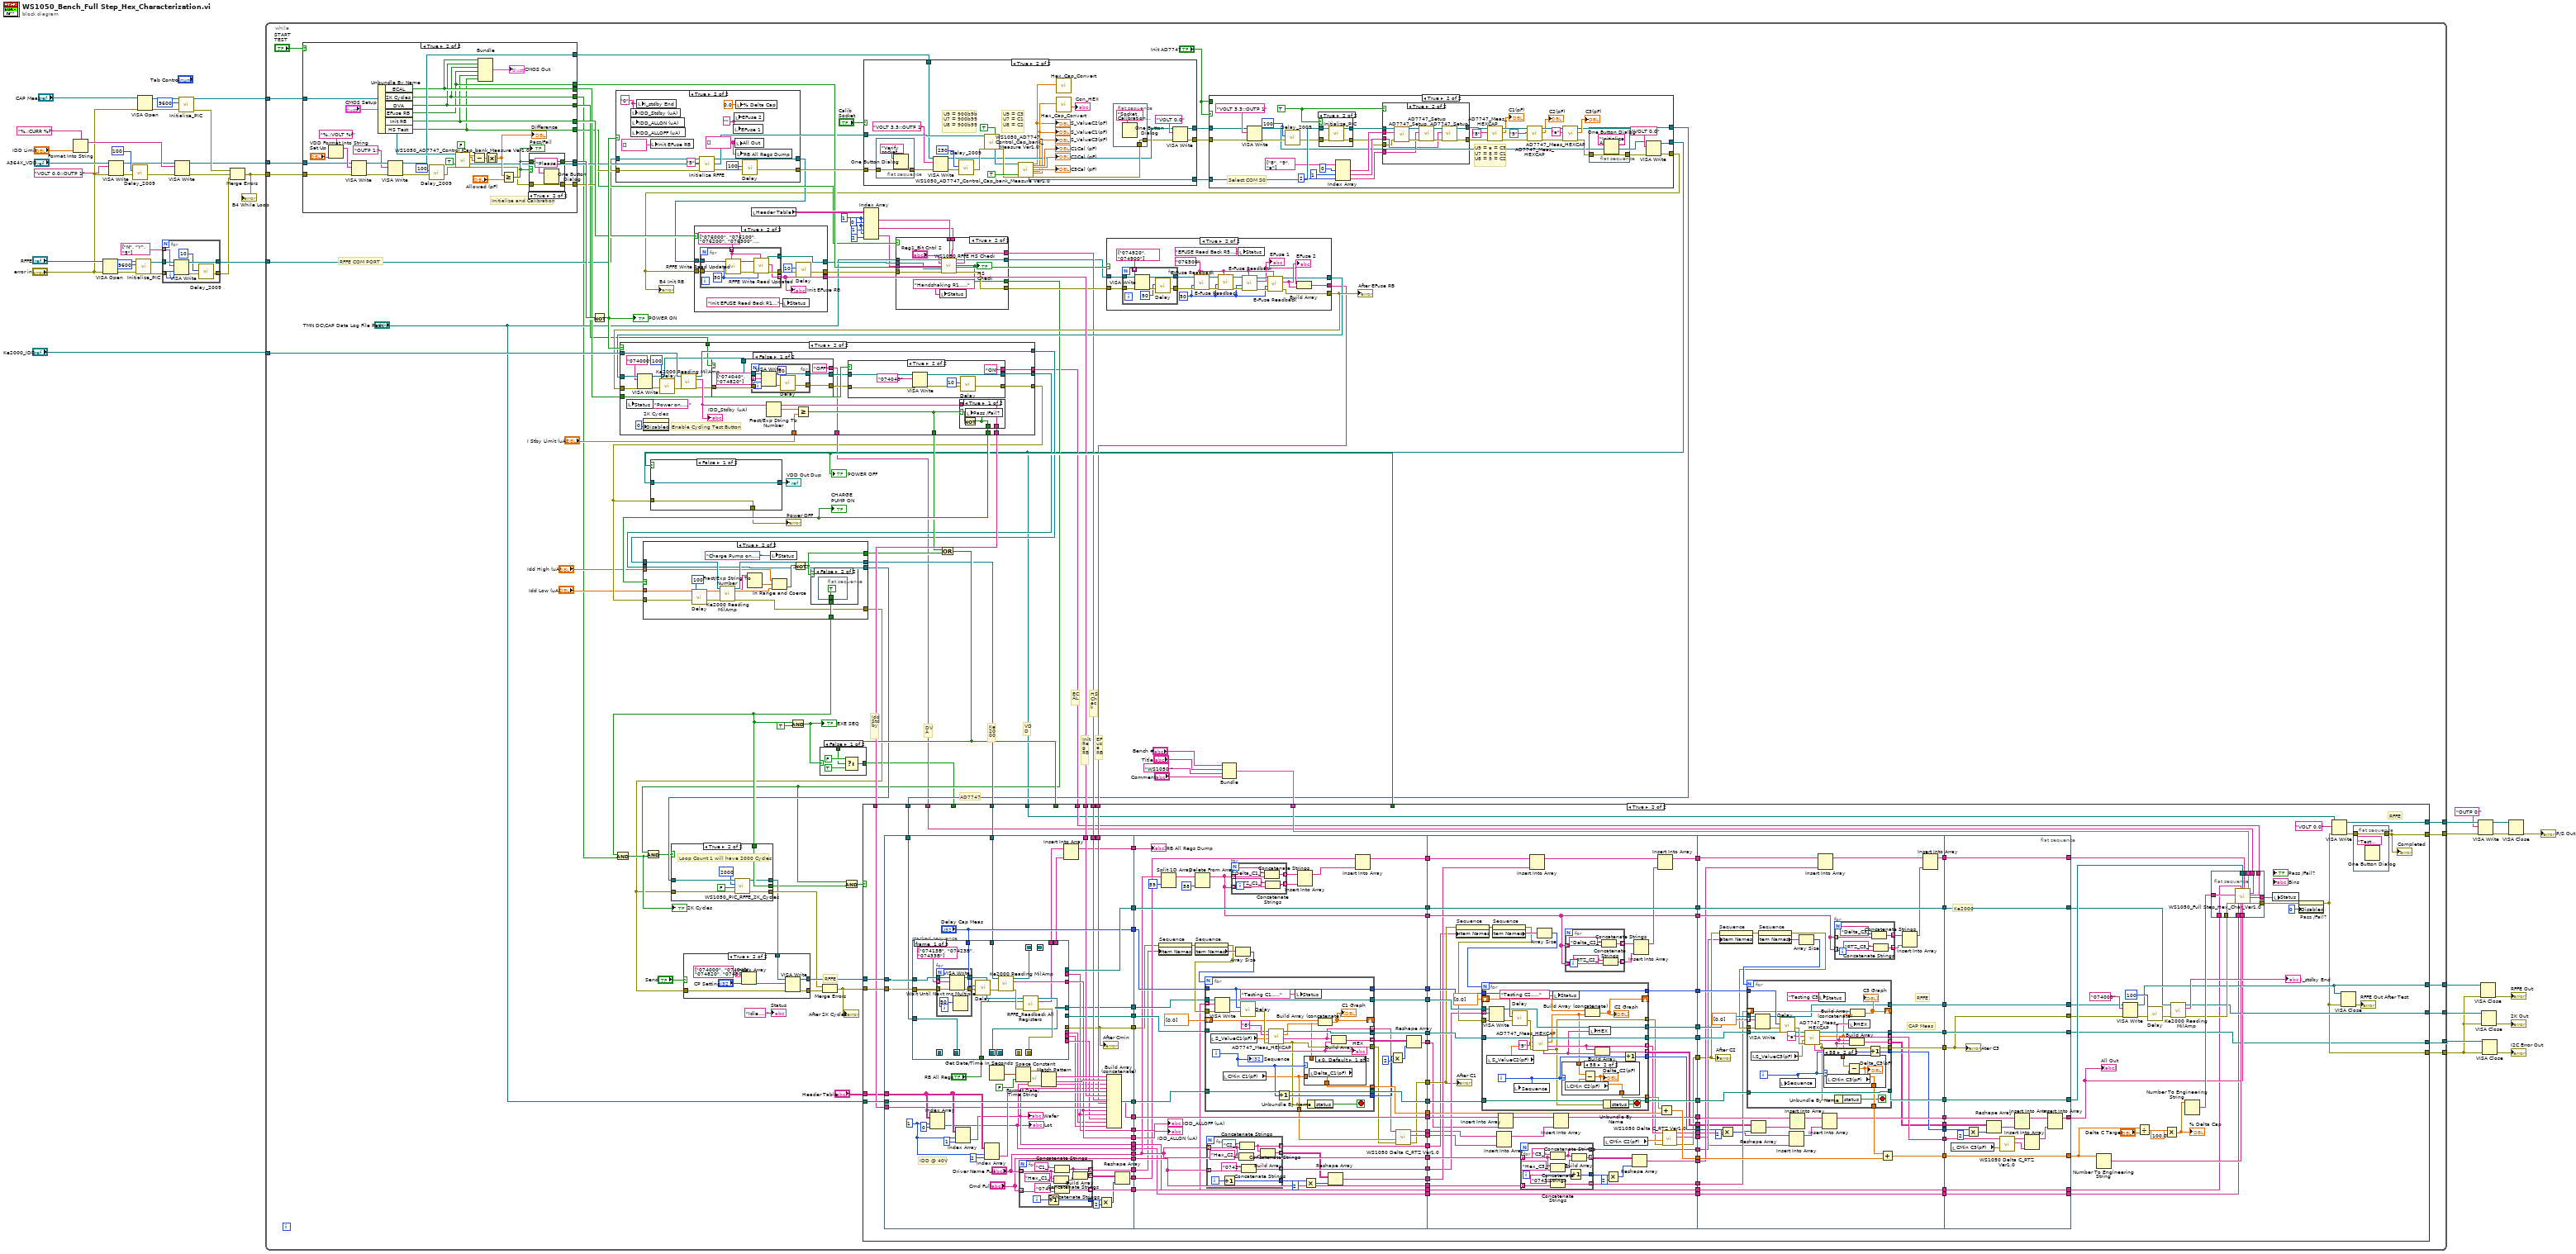
[diagram p0: block diagram]
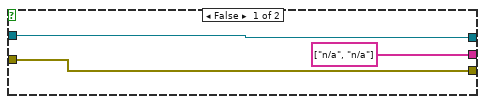
[diagram p2: hidden frame]
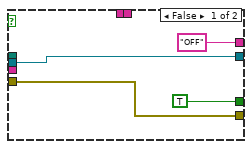
[diagram p3: hidden frame]
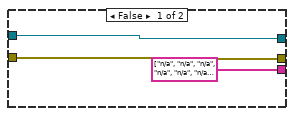
[diagram p4: hidden frame]
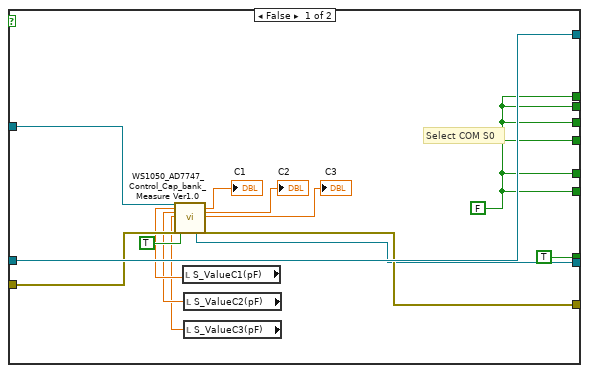
[diagram p11: hidden frame]
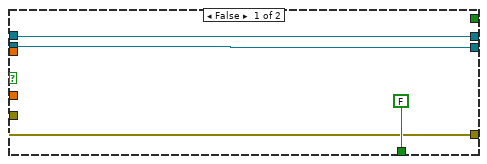
[diagram p15: hidden frame]
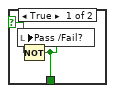
[diagram p16: hidden frame]
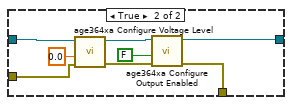
[diagram p17: hidden frame]
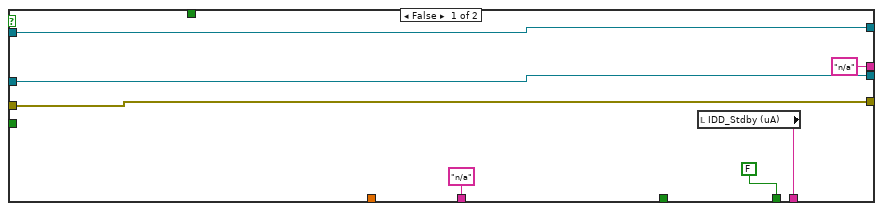
[diagram p18: hidden frame]
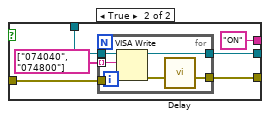
[diagram p19: hidden frame]
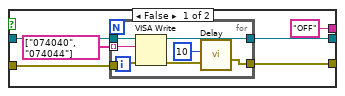
[diagram p20: hidden frame]
diagram:
  n1 = Format Into String(format string="%.;CURR %f", "IDD Limit") -> (resulting string=w12:string)  [unwired: 2 in, 1 out]
  n2 = VISA Open(error in (no error)="error in", VISA resource name="RFFE") -> (VISA resource name=w36:refnum<visa-resource-name>, error out=w35:errorcluster)  [unwired: 3 in]
  n3 = VISA Write(VISA resource name="A364X_VDD", write buffer="VOLT 0.0;:OUTP 1", error in (no error)="error in") -> (VISA resource name out=w11:refnum<visa-resource-name>, error out=w15:errorcluster)  [unwired: 1 out]
  n4 = call "Delay_2009.vi"("error in (no error)"=w15, "milliseconds to wait"=u32 100) -> ("error out"=w10:errorcluster)  [unwired: 9 in]
  n5 = call "Initialize_PIC.vi"("error in (no error)"=w35, "baud rate"=u32 9600, "Select Com Port"=w36) -> ("error out"=w34:errorcluster, "VISA resource name out"=w33:refnum<visa-resource-name>)  [unwired: 7 in]
  n6 = VISA Open(error in (no error)="error in", VISA resource name="CAP Meas") -> (VISA resource name=w39:refnum<visa-resource-name>, error out=w40:errorcluster)  [unwired: 3 in]
  n7 = for {
    tunnel: w34 -> [w49]
    tunnel: w33 -> [w48]
    tunnel: [w47] -> w31
    tunnel: [w45] -> w3
    tunnel: string[] ["N", "Y", "5"] -> [w43] mode=indexing
    n8 = VISA Write(VISA resource name=w48, write buffer=w43, error in (no error)=w49) -> (VISA resource name out=w47:refnum<visa-resource-name>, error out=w46:errorcluster)  [unwired: 1 out]
    n9 = call "Delay_2009.vi"("error in (no error)"=w46, "milliseconds to wait"=u32 10) -> ("error out"=w45:errorcluster)  [unwired: 9 in]
  }
  n10 = VISA Write(VISA resource name=w11, write buffer=w12, error in (no error)=w10) -> (VISA resource name out=w9:refnum<visa-resource-name>, error out=w8:errorcluster)  [unwired: 1 out]
  n11 = call "Initialize_PIC.vi"("error in (no error)"=w40, "baud rate"=u32 9600, "Select Com Port"=w39) -> ("error out"=w23:errorcluster, "VISA resource name out"=w32:refnum<visa-resource-name>)  [unwired: 7 in]
  n12 = Merge Errors(w23, w8, w3) -> (w42:errorcluster)
  "B4 While Loop" <- w42
  n13 = while {
    tunnel: [w136] -> w21
    tunnel: w32 -> [w85]
    tunnel: w9 -> [w117]
    tunnel: [w123] -> w20
    tunnel: [w121] -> w6
    tunnel: w42 -> [w73]
    tunnel: [w120] -> w41
    tunnel: "Ke2000_IDD" -> [w118]
    tunnel: [w94] -> w25
    tunnel: w31 -> [w70]
    tunnel: [w89] -> w28
    stop <- "CLICK DOWN TO QUIT" continue-if-true
    w55 = 1 ("index (row)")
    # "RFFE"
    # "Ke2000"
    # "Idd Stdby"
    # "Init Reg RB"
    # "HS Check"
    # "EFuse RB"
    # "ECAL"
    # "DVA"
    # "VDD"
    # "AD7747"
    # "RFFE COM PORT"
    n14 = case shown="True" "START \nTEST" {
      tunnel: [w332 w359] -> w104
      tunnel: [TRUE ("Pass/Fail") w366] -> w138
      tunnel: w85 -> [w331 w363]
      tunnel: w117 -> [w334 w349]
      tunnel: [w334 w344] -> w51
      tunnel: [w330 w360] -> w88
      tunnel: w73 -> [w333 w348]
      tunnel: [w322 w338] -> w108
      tunnel: [w322 w339] -> w93
      tunnel: [w322 w343] -> w81
      tunnel: [w322 w341] -> w63
      tunnel: [w322 w342] -> w80
      tunnel: [w322 w337] -> w71
      frame False {
        w322 = FALSE ("Initial E-Fuse")
        # "Select COM S0"
        n15 = local read "S_ValueC1(pF)"() -> (w328:dbl)
        n16 = local read "S_ValueC2(pF)"() -> (w327:dbl)
        n17 = local read "S_ValueC3(pF)"() -> (w326:dbl)
        n18 = call "WS1050_AD7747_Control_Cap_bank_Measure Ver1.0.vi"("Select Com Port"=w331, "S_Value C1"=w328, "S_Value C2"=w327, "S_Value C3"=w326, "errorin"=w333, "Push Button to Measue Cap"=TRUE) -> ("Com Port Out"=w330:refnum<visa-resource-name>, "C1_Mesa(pF)"=→"C1":dbl, "C2_Mesa(pF)"=→"C2":dbl, "C3_Mesa(pF)"=→"C3":dbl, "error out"=w332:errorcluster)  [unwired: 14 in, 3 out]
      }
      frame True {
        # "Initialize and Calibration"
        n19 = Format Into String(format string="%.;VOLT %f", "VDD \nSet Up") -> (resulting string=w350:string)  [unwired: 2 in, 1 out]
        n20 = VISA Write(VISA resource name=w349, write buffer=w350, error in (no error)=w348) -> (VISA resource name out=w346:refnum<visa-resource-name>, error out=w347:errorcluster)  [unwired: 1 out]
        n21 = Unbundle By Name("CMOS Setup") -> ("ECAL"=w343:bool, "2K Cycles"=w341:bool, "DVA"=w342:bool, "EFuse RB"=w339:bool, "Init RB"=w338:bool, "HS Test"=w337:bool)
        n22 = VISA Write(VISA resource name=w346, write buffer="OUTP 1;", error in (no error)=w347) -> (VISA resource name out=w344:refnum<visa-resource-name>, error out=w340:errorcluster)  [unwired: 1 out]
        n23 = call "Delay_2009.vi"("error in (no error)"=w340, "milliseconds to wait"=u32 100) -> ("error out"=w355:errorcluster)  [unwired: 9 in]
        n24 = call "WS1050_AD7747_Control_Cap_bank_Measure Ver1.0.vi"("Select Com Port"=w363, "errorin"=w355, "Push Button to Measue Cap"=TRUE, "Mode"=FALSE) -> ("Com Port Out"=w360:refnum<visa-resource-name>, "C1_Mesa(pF)"=w358:dbl, "C2_Mesa(pF)"=w357:dbl, "error out"=w362:errorcluster)  [unwired: 16 in, 4 out]
        n25 = Subtract(x=w358, y=w357) -> (x-y=w361:dbl)
        n26 = Bundle("ECAL"=w343, "DVA"=w342, "2K Cycles"=w341, "EFuse RB"=w339, "Init RB"=w338, "HS Test"=w337) -> (→"CMOS Out":T2)  [unwired: 1 in]
        n27 = Absolute Value(x=w361) -> (abs(x)=w364:dbl)
        "Difference" <- w364
        n28 = Greater Or Equal?(x=w364, y="Allowed (pF)") -> (x >= y?=w367:bool)
        "Pass/Fail" <- w367
        n29 = case shown="True" w367 {
          tunnel: [w369 w372] -> w366
          tunnel: w367 -> [w369 w372]
          tunnel: w362 -> [w370 w371]
          tunnel: [w370 w371] -> w359
          frame False {
          }
          frame True {
            n30 = One Button Dialog(message="Please reinstall part") -> ()  [unwired: 1 in, 1 out]
          }
        }
      }
    }
    n31 = Not(x=w138) -> (.not. x?=w133:bool)
    "POWER ON" <- w133
    n32 = case shown="True" w133 {
      tunnel: w104 -> [w309 w312]
      tunnel: [w309 w317] -> w107
      tunnel: w70 -> [w308 w313]
      tunnel: [w308 w314] -> w69
      frame False {
      }
      frame True {
        w310 = string[] [] ("All Out")
        w320 = "" ("EFuse 2")
        w318 = "0" ("Idd_Standby")
        n33 = local write "IDD_Stdby (uA)"(w318) -> ()
        n34 = local write "IDD_ALLON (uA)"(w318) -> ()
        n35 = local write "IDD_ALLOFF (uA)"(w318) -> ()
        n36 = local write "I_stdby End"(w318) -> ()
        n37 = local write "Init EFuse RB"(string[] []) -> ()
        n38 = call "Initialize RFFE.vi"("error in (no error)"=w312, "write buffer"="5", "Select Com Port"=w313) -> ("error out"=w316:errorcluster, "VISA resource name out"=w314:refnum<visa-resource-name>)  [unwired: 7 in]
        n39 = local write "EFuse 1"(w320) -> ()
        n40 = local write "EFuse 2"(w320) -> ()
        n41 = local write "All Out"(w310) -> ()
        n42 = local write "% Delta Cap"(0.0 ("% Delta Cap")) -> ()
        n43 = local write "RB All Regs Dump"(w310) -> ()
        n44 = call "Delay.vi"("error in (no error)"=w316, "milliseconds to wait"=u32 100) -> ("error out"=w317:errorcluster)  [unwired: 9 in]
      }
    }
    n45 = local read "Header Table"() -> (w98:string[][])
    n46 = Index Array(array=w98, index (row) #1=w55, index (col) #1=0 ("disabled index (col)"), index (row) #2=w55, index (col) #2=1 ("disabled index (col)"), index (row) #3=w55, index (col) #3=2 ("disabled index (col)")) -> (element #1=w99:string, element #2=w56:string, element #3=w53:string)
    n47 = case shown="True" "Calib\nSocket" {
      tunnel: w107 -> [w277 w302]
      tunnel: [w277 w282] -> w124
      tunnel: w88 -> [w276 w303]
      tunnel: w51 -> [w275 w288]
      tunnel: [w275 w283] -> w52
      tunnel: [w276 w299] -> w122
      frame False {
      }
      frame True {
        # "U9 = 900b9b\nU7 = 900b99\nU8 = 900b99"
        # "U9 = C3\nU7 = C1\nU8 = C2"
        n48 = flat-sequence {
          tunnel: [w305] -> w289
          tunnel: w302 -> [w305]
          frame #0 {
            n49 = One Button Dialog(message="Verify socket should be empty") -> ()  [unwired: 1 in, 1 out]
          }
        }
        n50 = VISA Write(VISA resource name=w288, write buffer="VOLT 3.3;:OUTP 1", error in (no error)=w289) -> (VISA resource name out=w284:refnum<visa-resource-name>, error out=w286:errorcluster)  [unwired: 1 out]
        n51 = call "Delay_2009.vi"("error in (no error)"=w286, "milliseconds to wait"=u32 250) -> ("error out"=w291:errorcluster)  [unwired: 9 in]
        n52 = call "WS1050_AD7747_Control_Cap_bank_Measure Ver1.0.vi"("Select Com Port"=w303, "errorin"=w291, "Push Button to Calibrate"=TRUE ("Push Button to Initialize AD7747")) -> ("Com Port Out"=w296:refnum<visa-resource-name>, "error out"=w297:errorcluster)  [unwired: 17 in, 6 out]
        n53 = call "WS1050_AD7747_Control_Cap_bank_Measure Ver1.0.vi"("Select Com Port"=w296, "errorin"=w297, "Push Button to Measue Cap"=TRUE) -> ("Com Port Out"=w299:refnum<visa-resource-name>, "C2(pF)"=w278:dbl, "C1_Mesa(pF)"=→"C1Cal (pF)":dbl, "C2_Mesa(pF)"=→"C2Cal (pF)":dbl, "C3_Mesa(pF)"=→"C3Cal (pF)":dbl, "C1(pF)"=w280:dbl, "C3(pF)"=→"S_ValueC3(pF)":dbl, "error out"=w300:errorcluster)  [unwired: 17 in]
        "S_ValueC2(pF)" <- w278
        "S_ValueC1(pF)" <- w280
        n54 = call "Hex_Cap_Convert.vi"("CAP-Hex(pF)"=w280) -> ("Con_HEX"=→"Con_HEX":string)  [unwired: 5 in, 5 out]
        n55 = call "Hex_Cap_Convert.vi"("CAP-Hex(pF)"=w278) -> ()  [unwired: 5 in, 6 out]
        n56 = flat-sequence {
          tunnel: [w306] -> w281
          tunnel: w300 -> [w306]
          frame #0 {
            n57 = One Button Dialog(message="Socket Calibration Completed, Please insert DUT into the Socket") -> ()  [unwired: 1 in, 1 out]
          }
        }
        n58 = VISA Write(VISA resource name=w284, write buffer="VOLT 0.0", error in (no error)=w281) -> (VISA resource name out=w283:refnum<visa-resource-name>, error out=w282:errorcluster)  [unwired: 1 out]
      }
    }
    n59 = case shown="True" "Init AD7747" {
      tunnel: w122 -> [w216 w253]
      tunnel: [w217 w219] -> w50
      tunnel: w124 -> [w217 w224]
      tunnel: [w216 w229] -> w90
      tunnel: w52 -> [w215 w225]
      tunnel: [w215 w220] -> w76
      tunnel: "Init AD7747" -> [_ _]
      frame False {
      }
      frame True {
        w231 = TRUE
        # "Select COM S0"
        # "U9 = a = C3\nU7 = 8 = C1\nU8 = 9 = C2"
        n60 = VISA Write(VISA resource name=w225, write buffer="VOLT 3.3;:OUTP 1", error in (no error)=w224) -> (VISA resource name out=w221:refnum<visa-resource-name>, error out=w223:errorcluster)  [unwired: 1 out]
        n61 = call "Delay_2009.vi"("error in (no error)"=w223, "milliseconds to wait"=u32 100) -> ("error out"=w227:errorcluster)  [unwired: 9 in]
        n62 = case shown="True" w231 {
          tunnel: [w267 w272] -> w242
          tunnel: [w268 w271] -> w252
          tunnel: w253 -> [w268 w270]
          tunnel: w227 -> [w267 w269]
          frame False {
          }
          frame True {
            n63 = call "Initialize_PIC.vi"("error in (no error)"=w269, "Select Com Port"=w270) -> ("error out"=w272:errorcluster, "VISA resource name out"=w271:refnum<visa-resource-name>)  [unwired: 8 in]
          }
        }
        n64 = Index Array(array=string[] ["8", "9", "a"], index #1=0 ("index"), index #2=1 ("index"), index #3=2 ("index")) -> (element #1=w245:string, element #2=w244:string, element #3=w243:string)
        n65 = case shown="True" w231 {
          tunnel: w242 -> [w255 w258]
          tunnel: [w255 w256] -> w247
          tunnel: w252 -> [w254 w266]
          tunnel: w245 -> [_ w261]
          tunnel: w243 -> [_ w260]
          tunnel: w244 -> [_ w259]
          tunnel: [w254 w257] -> w246
          frame False {
          }
          frame True {
            n66 = call "AD7747_Setup.vi"("error in"=w258, "AD7747_Number"=w261, "Control"=w266) -> ("error out"=w265:errorcluster, "Control out"=w264:refnum<visa-resource-name>)  [unwired: 6 in, 1 out]
            n67 = call "AD7747_Setup.vi"("error in"=w265, "AD7747_Number"=w260, "Control"=w264) -> ("error out"=w263:errorcluster, "Control out"=w262:refnum<visa-resource-name>)  [unwired: 6 in, 1 out]
            n68 = call "AD7747_Setup.vi"("error in"=w263, "AD7747_Number"=w259, "Control"=w262) -> ("error out"=w256:errorcluster, "Control out"=w257:refnum<visa-resource-name>)  [unwired: 6 in, 1 out]
          }
        }
        n69 = call "AD7747_Meas_HEXCAP.vi"("error in (no error)"=w247, "AD7747_Number"="8", "Control"=w246) -> ("error"=w239:errorcluster, "CAP (pF)"=→"C1(pF)":dbl, "Control out"=w238:refnum<visa-resource-name>)  [unwired: 3 in, 3 out]
        n70 = call "AD7747_Meas_HEXCAP.vi"("error in (no error)"=w239, "AD7747_Number"="9", "Control"=w238) -> ("error"=w236:errorcluster, "CAP (pF)"=→"C2(pF)":dbl, "Control out"=w235:refnum<visa-resource-name>)  [unwired: 3 in, 3 out]
        n71 = call "AD7747_Meas_HEXCAP.vi"("error in (no error)"=w236, "AD7747_Number"="a", "Control"=w235) -> ("error"=w230:errorcluster, "CAP (pF)"=→"C3(pF)":dbl, "Control out"=w229:refnum<visa-resource-name>)  [unwired: 3 in, 3 out]
        n72 = flat-sequence {
          tunnel: w230 -> [w273]
          tunnel: [w273] -> w218
          frame #0 {
            n73 = One Button Dialog(message="Initialize AD7747 completed!") -> ()  [unwired: 1 in, 1 out]
          }
        }
        n74 = VISA Write(VISA resource name=w221, write buffer="VOLT 0.0", error in (no error)=w218) -> (VISA resource name out=w220:refnum<visa-resource-name>, error out=w219:errorcluster)  [unwired: 1 out]
      }
    }
    "B4 Init RB" <- w50
    n75 = case shown="True" w108 {
      tunnel: [string[] ["n/a", "n/a", "n/a", "n/a", "n/a", "n/a", "n/a", "n/a", "n/a", "n/a"] w196] -> w106
      tunnel: w50 -> [w191 w193]
      tunnel: [w191 w200] -> w67
      tunnel: w69 -> [w189 w192]
      tunnel: [w189 w198] -> w92
      frame False {
      }
      frame True {
        n76 = for {
          tunnel: w193 -> [w203]
          tunnel: w192 -> [w202]
          tunnel: [w207] -> w198
          tunnel: [w208] -> w196 mode=indexing
          tunnel: string[] ["076000", "076100", "076200", "076300", "076400", "076500", "076600", "076700", "076800", "076900"] -> [w201] mode=indexing
          tunnel: [w209] -> w194
          w204 = u32 50 ("delay before read (ms)")
          n77 = call "RFFE Write Read Updated.vi"("VISA resource name"=w202, "write buffer"=w201, "delay before read (ms)"=w204, "error in (no error)"=w203) -> ("VISA resource name out"=w206:refnum<visa-resource-name>, "error out"=w205:errorcluster)  [unwired: 4 in, 1 out]
          n78 = call "RFFE Write Read Updated.vi"("VISA resource name"=w206, "write buffer"=w201, "delay before read (ms)"=w204, "error in (no error)"=w205) -> ("VISA resource name out"=w207:refnum<visa-resource-name>, "EFuse Read Back"=w208:string, "error out"=w209:errorcluster)  [unwired: 4 in]
        }
        "Init EFuse RB" <- w196
        n79 = local write "Status"("Init EFUSE Read Back R1..." ("Status")) -> ()
        n80 = call "Delay.vi"("error in (no error)"=w194, "milliseconds to wait"=u32 10) -> ("error out"=w200:errorcluster)  [unwired: 9 in]
      }
    }
    n81 = case shown="True" w71 {
      tunnel: w67 -> [w176 w188]
      tunnel: [w176 w187] -> w103
      tunnel: "TMN DC\\CAP Data Log File Path" -> [_ w186]
      tunnel: ["OFF" w184] -> w97
      tunnel: w99 -> [_ w183]
      tunnel: w56 -> [_ w182]
      tunnel: w53 -> [_ w180]
      tunnel: w92 -> [w174 w179]
      tunnel: [w174 w178] -> w91
      tunnel: [TRUE ("P/F") w177] -> w82
      frame False {
      }
      frame True {
        n82 = local write "Status"("Handshaking R1....." ("Status")) -> ()
        n83 = call "WS1050 RFFE HS Check.vi"("file path (use dialog)"=w186, "Lot #"=w183, "Wafer #"=w182, "Reg1_Bit Cntrl"="Reg1_Bit Cntrl 2", "SN #"=w180, "RFFE COM Port"=w179, "error"=w188) -> ("VISA resource name out"=w178:refnum<visa-resource-name>, "s? t:f"=w184:string, "P/F"=w177:bool, "error out"=w187:errorcluster)  [unwired: 4 in, 1 out]
        "HS \nCheck" <- w177
      }
    }
    n84 = case shown="True" w93 {
      tunnel: [string[] ["n/a", "n/a"] w161] -> w96
      tunnel: w103 -> [w146 w165]
      tunnel: [w146 w148] -> w102
      tunnel: w91 -> [w144 w163]
      tunnel: [w144 w147] -> w101
      frame False {
      }
      frame True {
        w149 = u32 50 ("delay before read (ms)")
        w152 = "076500" ("write buffer")
        n85 = for {
          tunnel: w165 -> [w172]
          tunnel: string[] ["074920", "074900"] -> [w171] mode=indexing
          tunnel: w163 -> [w170]
          tunnel: [w167] -> w159
          tunnel: [w169] -> w160
          n86 = VISA Write(VISA resource name=w170, write buffer=w171, error in (no error)=w172) -> (VISA resource name out=w169:refnum<visa-resource-name>, error out=w168:errorcluster)  [unwired: 1 out]
          n87 = call "Delay.vi"("error in (no error)"=w168, "milliseconds to wait"=u32 50) -> ("error out"=w167:errorcluster)  [unwired: 9 in]
        }
        n88 = call "E-Fuse Readback.vi"("write buffer"=w152, "error in (no error)"=w159, "delay before read (ms)"=w149, "VISA resource name"=w160) -> ("error out"=w158:errorcluster, "VISA resource name out"=w157:refnum<visa-resource-name>)  [unwired: 5 in, 1 out]
        n89 = call "E-Fuse Readback.vi"("write buffer"=w152, "error in (no error)"=w158, "delay before read (ms)"=w149, "VISA resource name"=w157) -> ("error out"=w156:errorcluster, "VISA resource name out"=w155:refnum<visa-resource-name>)  [unwired: 5 in, 1 out]
        n90 = local write "Status"("EFUSE Read Back R5....." ("Status")) -> ()
        n91 = call "E-Fuse Readback.vi"("write buffer"=w152, "error in (no error)"=w156, "delay before read (ms)"=w149, "VISA resource name"=w155) -> ("error out"=w154:errorcluster, "EFuse Read Back"=w150:string, "VISA resource name out"=w153:refnum<visa-resource-name>)  [unwired: 5 in]
        "EFuse 1" <- w150
        n92 = call "E-Fuse Readback.vi"("write buffer"=w152, "error in (no error)"=w154, "delay before read (ms)"=w149, "VISA resource name"=w153) -> ("error out"=w148:errorcluster, "EFuse Read Back"=w151:string, "VISA resource name out"=w147:refnum<visa-resource-name>)  [unwired: 5 in]
        "EFuse 2" <- w151
        n93 = Build Array(w150, w151) -> (w161:string[])
      }
    }
    "After EFuse RB" <- w102
    n94 = case shown="True" w133 {
      tunnel: [w432 w455] -> w139
      tunnel: [FALSE ("Measure after Action?") w457] -> w137
      tunnel: [_ w458] -> w134
      tunnel: w102 -> [w430 w447]
      tunnel: [w430 w441] -> w68
      tunnel: w101 -> [w429 w445]
      tunnel: w118 -> [w428 w452]
      tunnel: [w429 w448] -> w116
      tunnel: [w428 w451] -> w115
      tunnel: w81 -> [_ w442]
      tunnel: w80 -> [_ w436]
      tunnel: ["n/a" w435] -> w79
      tunnel: ["n/a" w434] -> w78
      tunnel: "I Stby Limit (uA)" -> [_ w433]
      frame False {
        n95 = local read "IDD_Stdby (uA)"() -> (w432:string)
      }
      frame True {
        # "Enable Cycling Test Button"
        n96 = local write "Status"("Power on....." ("Status")) -> ()
        n97 = VISA Write(VISA resource name=w445, write buffer="074000", error in (no error)=w447) -> (VISA resource name out=w438:refnum<visa-resource-name>, error out=w446:errorcluster)  [unwired: 1 out]
        n98 = property on="2K Cycles" class="Bool"("Disabled"=u8 0) -> ()  [unwired: 2 in, 2 out]
        n99 = call "Delay.vi"("error in (no error)"=w446, "milliseconds to wait"=u32 100) -> ("error out"=w449:errorcluster)  [unwired: 9 in]
        n100 = call "Ke2000 Reading MilAmp.vi"("error in (no error)"=w449, "VISA resource name"=w452) -> ("error out"=w437:errorcluster, "uA"=w450:string, "VISA resource name out"=w451:refnum<visa-resource-name>)  [unwired: 7 in]
        "IDD_Stdby (uA)" <- w450
        n101 = case shown="False" w436 {
          tunnel: [w463 w477] -> w440
          tunnel: [w464 w476] -> w439
          tunnel: w438 -> [w462 w475]
          tunnel: w437 -> [w461 w474]
          tunnel: ["OFF" "ON"] -> w435
          frame False {
            n102 = for {
              tunnel: w462 -> [w471]
              tunnel: [w470] -> w464
              tunnel: w461 -> [w469]
              tunnel: [w467] -> w463
              tunnel: string[] ["074040", "074820"] -> [w466] mode=indexing
              n103 = VISA Write(VISA resource name=w471, write buffer=w466, error in (no error)=w469) -> (VISA resource name out=w470:refnum<visa-resource-name>, error out=w468:errorcluster)  [unwired: 1 out]
              n104 = call "Delay.vi"("error in (no error)"=w468, "milliseconds to wait"=u32 10) -> ("error out"=w467:errorcluster)  [unwired: 9 in]
            }
          }
          frame True {
            n105 = for {
              tunnel: w475 -> [w483]
              tunnel: [w482] -> w476
              tunnel: w474 -> [w481]
              tunnel: [w479] -> w477
              tunnel: string[] ["074040", "074800"] -> [w478] mode=indexing
              n106 = VISA Write(VISA resource name=w483, write buffer=w478, error in (no error)=w481) -> (VISA resource name out=w482:refnum<visa-resource-name>, error out=w480:errorcluster)  [unwired: 1 out]
              n107 = call "Delay.vi"("error in (no error)"=w480) -> ("error out"=w479:errorcluster)  [unwired: 10 in]
            }
          }
        }
        n108 = Fract/Exp String To Number(string=w450) -> (number=w453:dbl)  [unwired: 4 out]
        n109 = Greater Or Equal?(x=w453, y=w433) -> (x >= y?=w458:bool)
        n110 = case shown="True" w442 {
          tunnel: [w489 w499] -> w441
          tunnel: [w488 w504] -> w448
          tunnel: w440 -> [w487 w502]
          tunnel: w439 -> [w485 w501]
          tunnel: ["OFF" "ON"] -> w434
          frame False {
            n111 = for {
              tunnel: [w491] -> w489
              tunnel: w485 -> [w496]
              tunnel: [w495] -> w488
              tunnel: w487 -> [w494]
              tunnel: string[] ["074040", "074044"] -> [w493] mode=indexing
              n112 = VISA Write(VISA resource name=w496, write buffer=w493, error in (no error)=w494) -> (VISA resource name out=w495:refnum<visa-resource-name>, error out=w492:errorcluster)  [unwired: 1 out]
              n113 = call "Delay.vi"("error in (no error)"=w492, "milliseconds to wait"=u32 10) -> ("error out"=w491:errorcluster)  [unwired: 9 in]
            }
          }
          frame True {
            n114 = VISA Write(VISA resource name=w501, write buffer="074040", error in (no error)=w502) -> (VISA resource name out=w504:refnum<visa-resource-name>, error out=w498:errorcluster)  [unwired: 1 out]
            n115 = call "Delay.vi"("error in (no error)"=w498, "milliseconds to wait"=u32 10) -> ("error out"=w499:errorcluster)  [unwired: 9 in]
          }
        }
        n116 = case shown="True" w458 {
          selector: w458 -> [w507 _]
          tunnel: [w505 w510] -> w457
          tunnel: w450 -> [w506 w509]
          tunnel: [w506 w508] -> w455
          frame True {
            n117 = Not(x=w507) -> (.not. x?=w505:bool)
            n118 = local write "Pass /Fail?"(w505) -> ()
          }
          frame False {
            n119 = flat-sequence {
              tunnel: w509 -> [w512]
              tunnel: [w512] -> w508
              tunnel: [TRUE ("Pass/Fail")] -> w510
              frame #0 {
              }
            }
          }
        }
      }
    }
    "CHARGE \nPUMP ON" <- w137
    n120 = case shown="True" w137 {
      tunnel: [FALSE w411] -> w129
      tunnel: [_ w408] -> w135
      tunnel: "Idd Low (uA)" -> [_ w397]
      tunnel: w68 -> [w395 w400]
      tunnel: [w395 w403] -> w74
      tunnel: w116 -> [w393 w399]
      tunnel: w115 -> [w394 w405]
      tunnel: [w394 w404] -> w110
      tunnel: [w393 w399] -> w109
      tunnel: "Idd High (uA)" -> [_ w398]
      frame False {
      }
      frame True {
        n121 = call "Delay.vi"("error in (no error)"=w400, "milliseconds to wait"=u32 100) -> ("error out"=w407:errorcluster)  [unwired: 9 in]
        n122 = call "Ke2000 Reading MilAmp.vi"("error in (no error)"=w407, "VISA resource name"=w405) -> ("error out"=w403:errorcluster, "uA"=w401:string, "VISA resource name out"=w404:refnum<visa-resource-name>)  [unwired: 7 in]
        n123 = Fract/Exp String To Number(string=w401) -> (number=w402:dbl)  [unwired: 3 in, 1 out]
        n124 = local write "Status"("Charge Pump on....." ("Status")) -> ()
        n125 = In Range and Coerce(upper limit=w398, x=w402, lower limit=w397) -> (In Range?=w409:bool)  [unwired: 1 out]
        n126 = Not(x=w409) -> (.not. x?=w408:bool)
        n127 = case shown="False" w408 {
          selector: w408 -> [w413 _]
          tunnel: [w412 w414] -> w411
          frame True {
            n128 = Not(x=w413) -> (.not. x?=w412:bool)
            n129 = local write "Pass /Fail?"(w412) -> ()
          }
          frame False {
            n130 = flat-sequence {
              tunnel: [TRUE] -> w414
              frame #0 {
              }
            }
          }
        }
      }
    }
    n131 = And(x=w129, y=w63) -> (x .and. y?=w84:bool)
    "2K Cycles" <- w84
    n132 = Compound Arithmetic op=AND(w82, w84) -> (w83:bool)
    n133 = case shown="True" w83 {
      tunnel: [w376 w383] -> w87
      tunnel: w129 -> [w376 w383]
      tunnel: [w375 w381] -> w113
      tunnel: w74 -> [w375 w382]
      tunnel: w109 -> [w374 w378]
      tunnel: [w374 w380] -> w95
      frame False {
      }
      frame True {
        # "Loop Count 1 will have 2000 Cycles"
        n134 = call "WS1050_PIC_RFFE_2K_Cycles.vi"("error in (no error)"=w382, "Initialize"=FALSE, "Number of Cycles"=2000, "VISA resource name 2"=w378) -> ("error out"=w381:errorcluster, "VISA resource name out"=w380:refnum<visa-resource-name>)  [unwired: 5 in, 1 out]
      }
    }
    n135 = case shown="True" "Send" {
      tunnel: w95 -> [w384 w390]
      tunnel: w74 -> [w385 w389]
      tunnel: [w385 w387] -> w112
      tunnel: [w384 w386] -> w114
      frame False {
      }
      frame True {
        n136 = Index Array(array=string[] ["074000", "074040", "074820", "074800", "074044", "074040", "074776", "07476F", "074773", "07477B", "07477C", "074760", "074762", "074768", "07413B", "074100", "07423B", "074200", "07433B", "074300"], index="CP Setting") -> (element=w391:string)
        n137 = VISA Write(VISA resource name=w390, write buffer=w391, error in (no error)=w389) -> (VISA resource name out=w386:refnum<visa-resource-name>, error out=w387:errorcluster)  [unwired: 1 out]
      }
    }
    n138 = And(x=w129, y=TRUE) -> (x .and. y?=w128:bool)
    "EXE SEQ" <- w128
    n139 = Merge Errors(w113, w112) -> (w111:errorcluster)
    "After 2K Cycles" <- w111
    n140 = Compound Arithmetic op=AND(w82, w87) -> (w86:bool)
    n141 = Or(x=w134, y=w135) -> (x .or. y?=w127:bool)
    n142 = case shown="False" w128 {
      selector: w128 -> [_ w214]
      tunnel: [w211 w214] -> w62
      tunnel: w127 -> [w210 _]
      frame False {
        n143 = Select(t=FALSE ("status"), s=w210, f=TRUE ("status")) -> (s? t:f=w211:bool)
      }
      frame True {
      }
    }
    n144 = Bundle("Bench #"="Bench #", "Title"="Title", "string"="WS1050 ", "Comment"="Comment") -> (w125:T3)  [unwired: 1 in]
    n145 = case shown="True" w86 {
      tunnel: "TMN DC\\CAP Data Log File Path" -> [w530 w695]
      tunnel: w127 -> [w529 _]
      tunnel: w139 -> [w528 w671]
      tunnel: [w516 _] -> w130
      tunnel: [w515 w633] -> w136
      tunnel: w111 -> [w525 w691]
      tunnel: w62 -> [w527 _]
      tunnel: w125 -> [w526 w665]
      tunnel: [w520 w619] -> w123
      tunnel: [w515 w612] -> w121
      tunnel: [w518 w613] -> w120
      tunnel: w114 -> [w518 w680]
      tunnel: w110 -> [w517 w678]
      tunnel: w106 -> [w524 w657]
      tunnel: "Header Table" -> [w523 w664]
      tunnel: w97 -> [w522 w656]
      tunnel: w96 -> [w521 w655]
      tunnel: [w517 w654] -> w94
      tunnel: w90 -> [w519 w653]
      tunnel: [w519 w605] -> w89
      tunnel: w76 -> [w520 w607]
      tunnel: w79 -> [w513 w614]
      tunnel: w78 -> [w514 w615]
      frame False {
        n146 = case shown="False" w527 {
          tunnel: w530 -> [_ w545]
          tunnel: w529 -> [_ w544]
          tunnel: w528 -> [_ w537]
          tunnel: [FALSE ("Pass/Fail?") w543] -> w516
          tunnel: w526 -> [_ w542]
          tunnel: w525 -> [w531 w541]
          tunnel: [w531 w540] -> w515
          tunnel: w524 -> [_ w539]
          tunnel: w523 -> [_ w538]
          tunnel: w522 -> [_ w536]
          tunnel: w521 -> [_ w535]
          tunnel: w514 -> [_ w534]
          tunnel: w513 -> [_ w533]
          frame True {
          }
          frame False {
            n147 = case shown="True" w544 {
              tunnel: w545 -> [_ w577]
              tunnel: [TRUE ("Pass/Fail?") w574] -> w543
              tunnel: w542 -> [_ w567]
              tunnel: w541 -> [w546 w569]
              tunnel: [w546 w568] -> w540
              tunnel: w539 -> [_ w556]
              tunnel: w538 -> [_ w566]
              tunnel: w537 -> [_ w553]
              tunnel: w536 -> [_ w555]
              tunnel: w535 -> [_ w554]
              tunnel: w534 -> [_ w549]
              tunnel: w533 -> [_ w548]
              frame False {
              }
              frame True {
                w550 = "na" ("Total Delta C")
                w560 = 1 ("index (row)")
                n148 = Get Date/Time In Seconds() -> (seconds since 1Jan1904=w573:timestamp)
                n149 = Format Date/Time String(seconds (now)=w573, UTC format=FALSE) -> (date/time string=w571:string)  [unwired: 1 in]
                n150 = call <vilib>:"Space Constant.vi"() -> ("String"=w570:string)
                n151 = Index Array(array=w566, index (row) #1=w560, index (col) #1=0 ("index (row)"), index (row) #2=w560, index (col) #2=1 ("index (row)"), index (row) #3=w560, index (col) #3=2 ("disabled index (col)")) -> (element #1=w563:string, element #2=w562:string, element #3=w561:string)
                n152 = Match Pattern(string=w571, regular expression=w570) -> (before substring=w565:string, after substring=w564:string)  [unwired: 1 in, 2 out]
                n153 = for {
                  N: 708 -> [_]
                  tunnel: ["na" ("new element/subarray")] -> w551 mode=indexing
                }
                n154 = Build Array (concatenate)(w565, w564, w563, w562, w561, w556, w555, w554, w553) -> (w558:string[])
                n155 = Insert Into Array(array=w558, new element=w551) -> (w557:string[])  [unwired: 1 in]
                n156 = call "WS1050_Full Step_Hex_Char_Ver1.0.vi"("% Delta C"=w550, "error in (no error)"=w569, "Lot"=w563, "Wafer"=w562, "Total Delta C"=w550, "TMN DC\\CAP Data Log File Path"=w577, "All Out"=w557, "Test Program"=w567, "DVA"=w548, "ECAL"=w549) -> ("error out"=w568:errorcluster)  [unwired: 15 in, 2 out]
                n157 = flat-sequence {
                  tunnel: [TRUE ("Pass/Fail?")] -> w574
                  frame #0 {
                  }
                }
              }
            }
          }
        }
      }
      frame True {
        # "RFFE"
        n158 = flat-sequence {
          tunnel: w691 -> [w735]
          tunnel: w695 -> [w757]
          tunnel: [w757] -> w682
          tunnel: [w719] -> w681
          tunnel: w680 -> [w736]
          tunnel: [w737] -> w679
          tunnel: w678 -> [w754]
          tunnel: [w756] -> w676
          tunnel: ["Delay Cap Meas"] -> w674
          tunnel: [w753] -> w673
          tunnel: w671 -> [w726]
          tunnel: w664 -> [w741]
          tunnel: w657 -> [w740]
          tunnel: w656 -> [w739]
          tunnel: w655 -> [w738]
          tunnel: w653 -> [w734]
          tunnel: [w720] -> w652
          tunnel: [w718] -> w648
          tunnel: [w733] -> w646
          tunnel: ["Driver Name Full"] -> w645
          tunnel: ["Cmd Full"] -> w644
          tunnel: [w725] -> w624
          tunnel: [w724] -> w623
          tunnel: [w729] -> w621
          tunnel: [w713] -> w602
          tunnel: [w712] -> w601
          tunnel: [w711] -> w592
          tunnel: [w886] -> w690
          tunnel: [w885] -> w689
          tunnel: [w884] -> w688
          tunnel: [w835] -> w687
          tunnel: w682 -> [w887]
          tunnel: w681 -> [w847]
          tunnel: w679 -> [w873]
          tunnel: [w881] -> w677
          tunnel: w676 -> [w881]
          tunnel: w674 -> [w880]
          tunnel: w673 -> [w879]
          tunnel: [w879] -> w672
          tunnel: [w875] -> w669
          tunnel: w652 -> [w874]
          tunnel: [w872] -> w651
          tunnel: w648 -> [w850]
          tunnel: [w853] -> w647
          tunnel: w646 -> [w849]
          tunnel: w645 -> [w869]
          tunnel: w644 -> [w870]
          tunnel: [w871] -> w643
          tunnel: [w869] -> w642
          tunnel: [w870] -> w641
          tunnel: [w862] -> w638
          tunnel: [w861] -> w635
          tunnel: w624 -> [w860]
          tunnel: w623 -> [w859]
          tunnel: w621 -> [w858]
          tunnel: w602 -> [w852]
          tunnel: w601 -> [w851]
          tunnel: [w852] -> w600
          tunnel: [w851] -> w599
          tunnel: w592 -> [w848]
          tunnel: [w846] -> w591
          tunnel: [w842] -> w584
          tunnel: [w838] -> w583
          tunnel: [w837] -> w582
          tunnel: w690 -> [w972]
          tunnel: w689 -> [w987]
          tunnel: w688 -> [w986]
          tunnel: w687 -> [w947]
          tunnel: [w982] -> w686
          tunnel: [w936] -> w685
          tunnel: [w981] -> w684
          tunnel: [w980] -> w683
          tunnel: w677 -> [w979]
          tunnel: [w979] -> w675
          tunnel: w672 -> [w978]
          tunnel: [w963] -> w670
          tunnel: w669 -> [w975]
          tunnel: [w974] -> w668
          tunnel: w651 -> [w973]
          tunnel: [w971] -> w650
          tunnel: w647 -> [w949]
          tunnel: w643 -> [w948]
          tunnel: w642 -> [w970]
          tunnel: w641 -> [w969]
          tunnel: [w952] -> w640
          tunnel: [w967] -> w639
          tunnel: w638 -> [w966]
          tunnel: [w960] -> w637
          tunnel: w635 -> [w957]
          tunnel: [w957] -> w634
          tunnel: w600 -> [w951]
          tunnel: w599 -> [w950]
          tunnel: [w951] -> w598
          tunnel: [w950] -> w597
          tunnel: w591 -> [w946]
          tunnel: [w945] -> w590
          tunnel: [w944] -> w588
          tunnel: [w943] -> w587
          tunnel: w584 -> [w942]
          tunnel: w583 -> [w941]
          tunnel: w582 -> [w940]
          tunnel: [w935] -> w581
          tunnel: [w934] -> w580
          tunnel: w686 -> [w1076]
          tunnel: w685 -> [w1045]
          tunnel: w684 -> [w1072]
          tunnel: w683 -> [w1071]
          tunnel: [w1061] -> w632
          tunnel: [w1070] -> w631
          tunnel: [w1069] -> w630
          tunnel: w675 -> [w1068]
          tunnel: [w1068] -> w629
          tunnel: w670 -> [w1067]
          tunnel: [w1057] -> w628
          tunnel: w668 -> [w1064]
          tunnel: [w1063] -> w627
          tunnel: w650 -> [w1062]
          tunnel: [w1060] -> w626
          tunnel: w640 -> [w1046]
          tunnel: w639 -> [w1044]
          tunnel: w637 -> [w1047]
          tunnel: [w1052] -> w625
          tunnel: w634 -> [w1055]
          tunnel: w598 -> [w1049]
          tunnel: w597 -> [w1048]
          tunnel: [w1049] -> w596
          tunnel: [w1048] -> w595
          tunnel: w590 -> [w1043]
          tunnel: [w1042] -> w589
          tunnel: w588 -> [w1039]
          tunnel: w587 -> [w1038]
          tunnel: [w1035] -> w586
          tunnel: [w1036] -> w585
          tunnel: w581 -> [w1034]
          tunnel: w580 -> [w1033]
          tunnel: [w1132] -> w649
          tunnel: [w1119] -> w603
          tunnel: [w1126] -> w605
          tunnel: [w1125] -> w609
          tunnel: [w1131] -> w636
          tunnel: [w1130] -> w622
          tunnel: [w1120] -> w604
          tunnel: [w1127] -> w606
          tunnel: w625 -> [w1131]
          tunnel: w626 -> [w1126]
          tunnel: w627 -> [w1132]
          tunnel: w628 -> [w1124]
          tunnel: w629 -> [w1125]
          tunnel: w630 -> [w1119]
          tunnel: w631 -> [w1130]
          tunnel: w632 -> [w1120]
          tunnel: w596 -> [w1118]
          tunnel: w595 -> [w1117]
          tunnel: [w1118] -> w593
          tunnel: [w1117] -> w594
          tunnel: w589 -> [w1116]
          tunnel: w586 -> [w1114]
          tunnel: w585 -> [w1111]
          frame #0 {
            w750 = 1 ("index (row)")
            # "IDD @ 40V"
            n159 = stacked-sequence {
              seq-local: [w781 _ _] -> [_ w803 _]
              seq-local: [w772 _ _] -> [_ w805 _]
              seq-local: [w774 _ _] -> [_ w806 _]
              seq-local: [_ w796 _] -> [_ _ w826]
              seq-local: [_ w794 _] -> [_ _ w821]
              seq-local: [_ w798 _] -> [_ _ w820]
              seq-local: [w770 _ _] -> [_ w792 _]
              seq-local: [_ w792 _] -> [_ _ w813]
              tunnel: w735 -> [w784 _ _]
              tunnel: [_ _ w823] -> w719
              tunnel: w754 -> [w783 _ _]
              tunnel: [w782 _ _] -> w725
              tunnel: [_ w804 _] -> w724
              tunnel: [_ _ w820] -> w756
              tunnel: w736 -> [w780 _ _]
              tunnel: "Delay Cap Meas" -> [w777 w800 _]
              tunnel: [_ _ w832] -> w723
              tunnel: [_ _ w831] -> w722
              tunnel: [_ _ w830] -> w721
              tunnel: [_ _ w822] -> w737
              tunnel: [_ _ w821] -> w720
              tunnel: w734 -> [w770 _ _]
              tunnel: "RB All Regs" -> [w771 w793 _]
              tunnel: [_ w791 _] -> w728
              tunnel: [w769 _ _] -> w727
              frame #0 {
                n160 = for {
                  tunnel: w784 -> [w790]
                  tunnel: [w789] -> w773
                  tunnel: w780 -> [w788]
                  tunnel: [w787] -> w778
                  tunnel: string[] ["07413B", "07423B", "07433B"] -> [w786] mode=indexing
                  n161 = VISA Write(VISA resource name=w788, write buffer=w786, error in (no error)=w790) -> (VISA resource name out=w789:refnum<visa-resource-name>, error out=w787:errorcluster)  [unwired: 1 out]
                  n162 = Wait Until Next ms Multiple(millisecond multiple=u32 50) -> ()  [unwired: 1 out]
                }
                n163 = call "Delay.vi"("error in (no error)"=w778, "milliseconds to wait"=w777) -> ("error out"=w779:errorcluster)  [unwired: 9 in]
                n164 = call "Ke2000 Reading MilAmp.vi"("error in (no error)"=w779, "VISA resource name"=w783) -> ("error out"=w775:errorcluster, "uA"=w782:string, "VISA resource name out"=w781:refnum<visa-resource-name>)  [unwired: 7 in]
                n165 = call "RFFE_Readback All Registers.vi"("error out"=w775, "RB All Regs"=w771, "VISA IN"=w773) -> ("error out 2"=w774:errorcluster, "ALL Regs RB"=w769:string[], "VISA OUT"=w772:refnum<visa-resource-name>)  [unwired: 6 in]
              }
              frame #1 {
                n166 = for {
                  tunnel: w806 -> [w812]
                  tunnel: w805 -> [w811]
                  tunnel: [w810] -> w795
                  tunnel: [w809] -> w801
                  tunnel: string[] ["074100", "074200", "074300"] -> [w807] mode=indexing
                  n167 = VISA Write(VISA resource name=w811, write buffer=w807, error in (no error)=w812) -> (VISA resource name out=w810:refnum<visa-resource-name>, error out=w809:errorcluster)  [unwired: 1 out]
                  n168 = Wait Until Next ms Multiple(millisecond multiple=u32 50) -> ()  [unwired: 1 out]
                }
                n169 = call "Delay.vi"("error in (no error)"=w801, "milliseconds to wait"=w800) -> ("error out"=w802:errorcluster)  [unwired: 9 in]
                n170 = call "Ke2000 Reading MilAmp.vi"("error in (no error)"=w802, "VISA resource name"=w803) -> ("error out"=w797:errorcluster, "uA"=w804:string, "VISA resource name out"=w798:refnum<visa-resource-name>)  [unwired: 7 in]
                n171 = call "RFFE_Readback All Registers.vi"("error out"=w797, "RB All Regs"=w793, "VISA IN"=w795) -> ("error out 2"=w796:errorcluster, "ALL Regs RB"=w791:string[], "VISA OUT"=w794:refnum<visa-resource-name>)  [unwired: 6 in]
              }
              frame #2 {
                n172 = local read "S_ValueC1(pF)"() -> (w816:dbl)
                n173 = local read "S_ValueC2(pF)"() -> (w815:dbl)
                n174 = local read "S_ValueC3(pF)"() -> (w814:dbl)
                n175 = call "AD7747_Meas_HEXCAP.vi"("error in (no error)"=w826, "OFFSet Cal"=w816, "AD7747_Number"="8", "Control"=w813) -> ("error"=w824:errorcluster, 1:"CAP (pF)"=w832:string, 2:"CAP (pF)"=→"CMin C1(pF)":dbl, "Control out"=w825:refnum<visa-resource-name>)  [unwired: 2 in, 2 out]
                n176 = call "AD7747_Meas_HEXCAP.vi"("error in (no error)"=w824, "OFFSet Cal"=w815, "AD7747_Number"="9", "Control"=w825) -> ("error"=w834:errorcluster, 1:"CAP (pF)"=w831:string, 2:"CAP (pF)"=→"CMin C2(pF)":dbl, "Control out"=w833:refnum<visa-resource-name>)  [unwired: 2 in, 2 out]
                n177 = call "AD7747_Meas_HEXCAP.vi"("error in (no error)"=w834, "OFFSet Cal"=w814, "AD7747_Number"="a", "Control"=w833) -> ("error"=w823:errorcluster, 1:"CAP (pF)"=w830:string, 2:"CAP (pF)"=→"CMin C3(pF)":dbl, "Control out"=w822:refnum<visa-resource-name>)  [unwired: 2 in, 2 out]
              }
            }
            "After Cmin" <- w719
            n178 = Index Array(array=w741, index (row)=w750, index (col)=0 ("disabled index (col)")) -> (element=w712:string)
            "Lot" <- w712
            n179 = Index Array(array=w741, index (row)=w750, index (col)=1) -> (element=w713:string)
            "Wafer" <- w713
            n180 = Index Array(array=w741, index (row)=w750, index (col)=2) -> (element=w748:string)
            n181 = Get Date/Time In Seconds() -> (seconds since 1Jan1904=w744:timestamp)
            n182 = Format Date/Time String(seconds (now)=w744, UTC format=FALSE) -> (date/time string=w745:string)  [unwired: 1 out]
            n183 = for {
              tunnel: "Driver Name Full" -> [w764] mode=indexing
              tunnel: [w761] -> w717 mode=indexing
              tunnel: "Cmd Full" -> [w766] mode=indexing
              tunnel: [w765] -> w733 mode=indexing
              tunnel: [w759] -> w716
              tunnel: [w758] -> w711 mode=indexing
              i -> [w760]
              n184 = Increment(x=w760) -> (x+1=w759:i32)
              n185 = Concatenate Strings("Hex_C1_" ("string"), w764) -> (w762:string)
              n186 = Concatenate Strings("C1_" ("string"), w764) -> (w758:string)
              n187 = Concatenate Strings("0741" ("string"), w766) -> (w765:string)
              n188 = Build Array(w758, w762) -> (w761:string[])
            }
            n189 = call <vilib>:"Space Constant.vi"() -> ("String"=w746:string)
            n190 = Match Pattern(string=w745, regular expression=w746) -> (before substring=w743:string, after substring=w742:string)  [unwired: 3 out]
            n191 = Insert Into Array(array=w727, new element=w728) -> (w729:string[])  [unwired: 1 in]
            n192 = Multiply(x=w716, y=2) -> (x*y=w714:i32)
            n193 = Build Array (concatenate)(w743, w742, w712, w713, w748, w740, w739, w738, w726, w725, w724, w723, w722, w721) -> (w753:string[])
            n194 = Reshape Array(w717, w714) -> (w718:string[])
          }
          frame #1 {
            n195 = property on="Sequence" class="LstBox (strict)"(error in=w847, "Item Names"=w848) -> (error out=w883:errorcluster)  [unwired: 1 in, 1 out]
            n196 = Split 1D Array(array=w869, index=59) -> (first subarray=w867:string[])  [unwired: 1 out]
            n197 = Delete From Array(array=w867, index=58) -> (array with subset deleted=w861:string[])  [unwired: 1 in, 1 out]
            n198 = property on="Sequence" class="LstBox (strict)"(error in=w883) -> (error out=w877:errorcluster, "Item Names"=w882:string[])  [unwired: 1 in, 1 out]
            n199 = for {
              tunnel: w869 -> [w900] mode=indexing
              tunnel: [w897] -> w857 mode=indexing
              tunnel: w870 -> [w902] mode=indexing
              tunnel: [w901] -> w871 mode=indexing
              tunnel: [w895] -> w856
              tunnel: [w894] -> w846 mode=indexing
              i -> [w896]
              n200 = Increment(x=w896) -> (x+1=w895:i32)
              n201 = Concatenate Strings("Hex_C2_" ("string"), w900) -> (w898:string)
              n202 = Concatenate Strings("C2_" ("string"), w900) -> (w894:string)
              n203 = Concatenate Strings("0742" ("string"), w902) -> (w901:string)
              n204 = Build Array(w894, w898) -> (w897:string[])
            }
            n205 = for {
              tunnel: w861 -> [w893] mode=indexing
              tunnel: [w892] -> w865 mode=indexing
              tunnel: w861 -> [w890] mode=indexing
              tunnel: [w888] -> w864 mode=indexing
              n206 = Concatenate Strings("Delta_C1_" ("string"), w893) -> (w892:string)
              n207 = Concatenate Strings("RTZ_C1_" ("string"), w890) -> (w888:string)
            }
            n208 = Array Size(array=w882) -> (size(s)=w878:i32)
            n209 = for {
              N: w878 -> [_]
              tunnel: w887 -> [w928]
              tunnel: [w928] -> w885
              tunnel: [w924] -> w886
              tunnel: w880 -> [w922]
              tunnel: [w922] -> w884
              tunnel: w849 -> [w927] mode=indexing
              tunnel: w874 -> [w926]
              tunnel: w877 -> [w925]
              tunnel: [w907] -> w836
              shift-right: [w918] -> _
              shift-left: dbl[] [0.0] -> [w919]
              tunnel: [w917] -> w875
              tunnel: w873 -> [w916]
              tunnel: [w915] -> w872
              tunnel: [w912] -> w841
              tunnel: [w909] -> w843 mode=indexing
              tunnel: [w910] -> w840 mode=indexing
              tunnel: [w906] -> w839
              i -> [w913]
              stop <- w908 stop-if-true
              n210 = local read "S_ValueC1(pF)"() -> (w914:dbl)
              n211 = VISA Write(VISA resource name=w926, write buffer=w927, error in (no error)=w925) -> (VISA resource name out=w915:refnum<visa-resource-name>, error out=w923:errorcluster)  [unwired: 1 out]
              n212 = local read "CMin C1(pF)"() -> (w906:dbl)
              n213 = call "Delay.vi"("error in (no error)"=w923, "milliseconds to wait"=w922) -> ("error out"=w921:errorcluster)  [unwired: 9 in]
              n214 = call "AD7747_Meas_HEXCAP.vi"("error in (no error)"=w921, "OFFSet Cal"=w914, "AD7747_Number"="8", "Control"=w916) -> ("error"=w907:errorcluster, 1:"CAP (pF)"=w910:string, 2:"CAP (pF)"=w905:dbl, "Control out"=w924:refnum<visa-resource-name>, "HEX"=w911:string)  [unwired: 2 in, 1 out]
              "HEX" <- w911
              n215 = Increment(x=w913) -> (x+1=w912:i32)
              n216 = local write "Status"("Testing C1....." ("Status")) -> ()
              n217 = case shown="0, Default" w913 {
                tunnel: w905 -> [_ w933]
                tunnel: [w930 w932] -> w917
                tunnel: w906 -> [_ w931]
                frame 0, Default {
                  n218 = local read "Delta_C1(pF)"() -> (w930:dbl)
                }
                frame 58 {
                  n219 = Subtract(x=w933, y=w931) -> (x-y=w932:dbl)
                  "Delta_C1(pF)" <- w932
                }
              }
              n220 = Unbundle By Name(w907) -> ("status"=w908:bool)
              n221 = Build Array (concatenate)(w919, w905) -> (w918:dbl[])
              "C1 Graph" <- w918
              n222 = Build Array(w910, w911) -> (w909:string[])
              "Sequence" <- w913
            }
            n223 = Insert Into Array(array=w865, new element=w864) -> (w863:string[])  [unwired: 1 in]
            n224 = Multiply(x=w856, y=2) -> (x*y=w854:i32)
            n225 = Reshape Array(w857, w854) -> (w853:string[])
            n226 = Insert Into Array(array=w850, new element=w863) -> (w862:string[])  [unwired: 1 in]
            n227 = Multiply(x=w841, y=2) -> (x*y=w845:i32)
            n228 = call "WS1050 Delta C_RTZ Ver1.0.vi"("error in (no error)"=w836, "CMin_C1"=w839, "Bank C1"=w840) -> ("error out"=w835:errorcluster, "C1_RTZ"=w838:string[], "Delta C(pF)"=w837:string[])  [unwired: 6 in]
            n229 = Reshape Array(w843, w845) -> (w842:string[])
            "IDD_ALLON (uA)" <- w860
            "IDD_ALLOFF (uA)" <- w859
            "RB All Regs Dump" <- w858
          }
          frame #2 {
            n230 = property on="Sequence" class="LstBox (strict)"(error in=w947, "Item Names"=w946) -> (error out=w984:errorcluster)  [unwired: 1 in, 1 out]
            n231 = property on="Sequence" class="LstBox (strict)"(error in=w984) -> (error out=w968:errorcluster, "Item Names"=w985:string[])  [unwired: 1 in, 1 out]
            n232 = Insert Into Array(array=w940, new element=w941) -> (w964:string[])  [unwired: 1 in]
            n233 = Insert Into Array(array=w978, new element=w942) -> (w965:string[])  [unwired: 1 in]
            n234 = for {
              tunnel: w970 -> [w1000] mode=indexing
              tunnel: [w997] -> w956 mode=indexing
              tunnel: w969 -> [w1002] mode=indexing
              tunnel: [w1001] -> w967 mode=indexing
              tunnel: [w995] -> w955
              tunnel: [w994] -> w945 mode=indexing
              i -> [w996]
              n235 = Concatenate Strings("C3_" ("string"), w1000) -> (w994:string)
              n236 = Concatenate Strings("0743" ("string"), w1002) -> (w1001:string)
              n237 = Concatenate Strings("Hex_C3_" ("string"), w1000) -> (w998:string)
              n238 = Increment(x=w996) -> (x+1=w995:i32)
              n239 = Build Array(w994, w998) -> (w997:string[])
            }
            n240 = Insert Into Array(array=w966, new element=w949) -> (w958:string[])  [unwired: 1 in]
            n241 = Array Size(array=w985) -> (size(s)=w983:i32)
            n242 = for {
              N: w983 -> [_]
              tunnel: w987 -> [w1027]
              tunnel: [w1027] -> w982
              tunnel: w986 -> [w1022]
              tunnel: [w1022] -> w981
              tunnel: w948 -> [w1026] mode=indexing
              tunnel: w973 -> [w1025]
              tunnel: [w1012] -> w943 mode=indexing
              tunnel: [w1006] -> w937
              tunnel: w968 -> [w1021]
              tunnel: [w1015] -> w980
              shift-right: [w1018] -> _
              shift-left: dbl[] [0.0] -> [w1019]
              tunnel: [w1017] -> w976
              tunnel: w972 -> [w1016]
              tunnel: [w1014] -> w971
              tunnel: [w1010] -> w944
              tunnel: [w1009] -> w938 mode=indexing
              i -> [w1011]
              stop <- w1007 stop-if-true
              n243 = local read "S_ValueC2(pF)"() -> (w1013:dbl)
              n244 = VISA Write(VISA resource name=w1025, write buffer=w1026, error in (no error)=w1021) -> (VISA resource name out=w1015:refnum<visa-resource-name>, error out=w1023:errorcluster)  [unwired: 1 out]
              n245 = call "Delay.vi"("error in (no error)"=w1023, "milliseconds to wait"=w1022) -> ("error out"=w1024:errorcluster)  [unwired: 9 in]
              n246 = local write "Sequence"(w1011) -> ()
              n247 = call "AD7747_Meas_HEXCAP.vi"("error in (no error)"=w1024, "OFFSet Cal"=w1013, "AD7747_Number"="9" ("CNTR2_AD7747"), "Control"=w1016) -> ("error"=w1006:errorcluster, 1:"CAP (pF)"=w1009:string, 2:"CAP (pF)"=w1005:dbl, "Control out"=w1014:refnum<visa-resource-name>, "HEX"=w1008:string)  [unwired: 2 in, 1 out]
              n248 = local write "Status"("Testing C2....." ("Status")) -> ()
              n249 = case shown="58" w1011 {
                tunnel: w1005 -> [_ w1032]
                tunnel: [w1029 w1031] -> w1017
                frame 0, Default {
                  n250 = local read "Delta_C2(pF)"() -> (w1029:dbl)
                }
                frame 58 {
                  n251 = local read "CMin C2(pF)"() -> (w1030:dbl)
                  n252 = Subtract(x=w1032, y=w1030) -> (x-y=w1031:dbl)
                  "Delta_C2(pF)" <- w1031
                }
              }
              n253 = Build Array (concatenate)(w1019, w1005) -> (w1018:dbl[])
              "C2 Graph" <- w1018
              n254 = local write "HEX"(w1008) -> ()
              n255 = Build Array(w1009, w1008) -> (w1012:string[])
              n256 = Unbundle By Name(w1006) -> ("status"=w1007:bool)
              n257 = Increment(x=w1011) -> (x+1=w1010:i32)
            }
            n258 = Insert Into Array(array=w965, new element=w964) -> (w963:string[])  [unwired: 1 in]
            n259 = for {
              tunnel: w957 -> [w993] mode=indexing
              tunnel: [w992] -> w961 mode=indexing
              tunnel: w957 -> [w990] mode=indexing
              tunnel: [w988] -> w962 mode=indexing
              n260 = Concatenate Strings("Delta_C2_" ("string"), w993) -> (w992:string)
              n261 = Concatenate Strings("RTZ_C2_" ("string"), w990) -> (w988:string)
            }
            n262 = local read "CMin C2(pF)"() -> (w939:dbl)
            n263 = Multiply(x=w955, y=2) -> (x*y=w953:i32)
            n264 = Reshape Array(w956, w953) -> (w952:string[])
            n265 = Insert Into Array(array=w961, new element=w962) -> (w959:string[])  [unwired: 1 in]
            n266 = Insert Into Array(array=w958, new element=w959) -> (w960:string[])  [unwired: 1 in]
            n267 = Add(x=w976, y=w975) -> (x+y=w974:dbl)
            n268 = call "WS1050 Delta C_RTZ Ver1.0.vi"("error in (no error)"=w937, "CMin_C1"=w939, "Bank C1"=w938) -> ("error out"=w936:errorcluster, "C1_RTZ"=w934:string[], "Delta C(pF)"=w935:string[])  [unwired: 6 in]
            "After C1" <- w947
          }
          frame #3 {
            # "RFFE"
            # "CAP Meas"
            n269 = property on="Sequence" class="LstBox (strict)"(error in=w1045, "Item Names"=w1043) -> (error out=w1075:errorcluster)  [unwired: 1 in, 1 out]
            n270 = Multiply(x=w1039, y=2) -> (x*y=w1040:i32)
            n271 = Reshape Array(w1038, w1040) -> (w1037:string[])
            n272 = property on="Sequence" class="LstBox (strict)"(error in=w1075) -> (error out=w1056:errorcluster, "Item Names"=w1074:string[])  [unwired: 1 in, 1 out]
            n273 = Insert Into Array(array=w1034, new element=w1033) -> (w1058:string[])  [unwired: 1 in]
            n274 = Insert Into Array(array=w1067, new element=w1037) -> (w1059:string[])  [unwired: 1 in]
            n275 = Array Size(array=w1074) -> (size(s)=w1073:i32)
            n276 = for {
              N: w1073 -> [_]
              tunnel: w1076 -> [w1105]
              tunnel: [w1105] -> w1070
              tunnel: w1072 -> [w1100]
              tunnel: w1044 -> [w1104] mode=indexing
              tunnel: w1071 -> [w1103]
              tunnel: [w1090] -> w1035 mode=indexing
              tunnel: [w1085] -> w1069
              tunnel: [w1098] -> w1060
              tunnel: w1056 -> [w1099]
              shift-right: [w1095] -> _
              shift-left: dbl[] [0.0] -> [w1096]
              tunnel: [w1094] -> w1065
              tunnel: w1062 -> [w1093]
              tunnel: [w1092] -> w1061
              tunnel: [w1088] -> w1036
              tunnel: [w1087] -> w1042 mode=indexing
              i -> [w1089]
              stop <- w1084 stop-if-true
              n277 = local read "S_ValueC3(pF)"() -> (w1091:dbl)
              n278 = VISA Write(VISA resource name=w1103, write buffer=w1104, error in (no error)=w1099) -> (VISA resource name out=w1092:refnum<visa-resource-name>, error out=w1101:errorcluster)  [unwired: 1 out]
              n279 = local write "Sequence"(w1089) -> ()
              n280 = call "Delay.vi"("error in (no error)"=w1101, "milliseconds to wait"=w1100) -> ("error out"=w1102:errorcluster)  [unwired: 9 in]
              n281 = call "AD7747_Meas_HEXCAP.vi"("error in (no error)"=w1102, "OFFSet Cal"=w1091, "AD7747_Number"="a" ("CNTR1_AD7747"), "Control"=w1093) -> ("error"=w1085:errorcluster, 1:"CAP (pF)"=w1087:string, 2:"CAP (pF)"=w1083:dbl, "Control out"=w1098:refnum<visa-resource-name>, "HEX"=w1086:string)  [unwired: 2 in, 1 out]
              n282 = local write "Status"("Testing C3....." ("Status")) -> ()
              n283 = case shown="58" w1089 {
                tunnel: w1083 -> [_ w1110]
                tunnel: [w1107 w1109] -> w1094
                frame 0, Default {
                  n284 = local read "Delta_C3(pF)"() -> (w1107:dbl)
                }
                frame 58 {
                  n285 = local read "CMin C3(pF)"() -> (w1108:dbl)
                  n286 = Subtract(x=w1110, y=w1108) -> (x-y=w1109:dbl)
                  "Delta_C3(pF)" <- w1109
                }
              }
              n287 = Unbundle By Name(w1085) -> ("status"=w1084:bool)
              n288 = local write "HEX"(w1086) -> ()
              n289 = Build Array(w1087, w1086) -> (w1090:string[])
              n290 = Build Array (concatenate)(w1096, w1083) -> (w1095:dbl[])
              "C3 Graph" <- w1095
              n291 = Increment(x=w1089) -> (x+1=w1088:i32)
            }
            n292 = Insert Into Array(array=w1047, new element=w1046) -> (w1050:string[])  [unwired: 1 in]
            n293 = Insert Into Array(array=w1059, new element=w1058) -> (w1057:string[])  [unwired: 1 in]
            n294 = for {
              tunnel: w1055 -> [w1082] mode=indexing
              tunnel: [w1081] -> w1053 mode=indexing
              tunnel: [w1078] -> w1054 mode=indexing
              tunnel: w1055 -> [w1077] mode=indexing
              n295 = Concatenate Strings("Delta_C3_" ("string"), w1082) -> (w1081:string)
              n296 = Concatenate Strings("RTZ_C3_" ("string"), w1077) -> (w1078:string)
            }
            n297 = Add(x=w1065, y=w1064) -> (x+y=w1063:dbl)
            n298 = Insert Into Array(array=w1053, new element=w1054) -> (w1051:string[])  [unwired: 1 in]
            n299 = Insert Into Array(array=w1050, new element=w1051) -> (w1052:string[])  [unwired: 1 in]
            "After C2" <- w1045
          }
          frame #4 {
            # "Ke2000"
            n300 = local read "CMin C3(pF)"() -> (w1121:dbl)
            n301 = Multiply(x=w1111, y=2 ("x")) -> (x*y=w1113:i32)
            n302 = Reshape Array(w1114, w1113) -> (w1115:string[])
            n303 = call "WS1050 Delta C_RTZ Ver1.0.vi"("CMin_C1"=w1121, "Bank C1"=w1116) -> ("C1_RTZ"=w1122:string[], "Delta C(pF)"=w1123:string[])  [unwired: 7 in, 1 out]
            n304 = Insert Into Array(array=w1124, new element=w1115) -> (w1129:string[])  [unwired: 1 in]
            n305 = Insert Into Array(array=w1123, new element=w1122) -> (w1128:string[])  [unwired: 1 in]
            n306 = Insert Into Array(array=w1129, new element=w1128) -> (w1127:string[])  [unwired: 1 in]
            "Ater C3" <- w1119
          }
        }
        n307 = Number To Engineering String(4:w649) -> (0:w666:string)  [unwired: 3 in]
        n308 = VISA Write(VISA resource name=w604, write buffer="074000", error in (no error)=w603) -> (VISA resource name out=w613:refnum<visa-resource-name>, error out=w662:errorcluster)  [unwired: 1 out]
        n309 = Divide(x=w649, y="Delta C Target") -> (x/y=w617:dbl)
        n310 = call "Delay.vi"("error in (no error)"=w662, "milliseconds to wait"=u32 100) -> ("error out"=w661:errorcluster)  [unwired: 9 in]
        n311 = Multiply(x=w617, y=100.0) -> (x*y=w608:dbl)
        "% Delta Cap" <- w608
        n312 = call "Ke2000 Reading MilAmp.vi"("error in (no error)"=w661, "VISA resource name"=w609) -> ("error out"=w658:errorcluster, "uA"=→"I_stdby End":string, "VISA resource name out"=w654:refnum<visa-resource-name>)  [unwired: 7 in]
        n313 = Number To Engineering String(4:w608) -> (0:w667:string)  [unwired: 3 in]
        n314 = flat-sequence {
          tunnel: [w708] -> w694
          tunnel: [w707] -> w692
          tunnel: w667 -> [w706]
          tunnel: w666 -> [w698]
          tunnel: w665 -> [w705]
          tunnel: w658 -> [w704]
          tunnel: w606 -> [w703]
          tunnel: w636 -> [w702]
          tunnel: w622 -> [w701]
          tunnel: w615 -> [w700]
          tunnel: w614 -> [w699]
          tunnel: w594 -> [w697]
          tunnel: w593 -> [w696]
          frame #0 {
            n315 = call "WS1050_Full Step_Hex_Char_Ver1.0.vi"("% Delta C"=w706, "error in (no error)"=w704, "Lot"=w697, "Wafer"=w696, "Total Delta C"=w698, "TMN DC\\CAP Data Log File Path"=w701, "All Out"=w703, "WS1050 CAP Header"=w702, "Test Program"=w705, "DVA"=w699, "ECAL"=w700) -> ("Status"=w708:string, "error out"=w707:errorcluster)  [unwired: 14 in, 1 out]
          }
        }
        n316 = local write "Status"(w694) -> ()
        n317 = property on="Pass /Fail?" class="Bool (strict)"(error in=w692, "Disabled"=u8 0) -> (error out=w612:errorcluster)  [unwired: 1 in, 1 out]
        n318 = VISA Write(VISA resource name=w607, write buffer="VOLT 0.0", error in (no error)=w612) -> (VISA resource name out=w619:refnum<visa-resource-name>, error out=w610:errorcluster)  [unwired: 1 out]
        n319 = VISA Close(VISA resource name=w613, error in (no error)=w612) -> (error out=→"RFFE Out After Test":errorcluster)
        n320 = flat-sequence {
          tunnel: w610 -> [w710]
          tunnel: [w710] -> w633
          frame #0 {
            n321 = One Button Dialog(message="Test Completed") -> ()  [unwired: 1 in, 1 out]
          }
        }
        "Completed" <- w633
        "All Out" <- w606
      }
    }
    "POWER OFF" <- w130
    n322 = case shown="False" w130 {
      tunnel: w68 -> [w417 w425]
      tunnel: [w417 w421] -> w77
      tunnel: w76 -> [w416 w419]
      tunnel: [w416 w418] -> w75
      frame False {
      }
      frame True {
        n323 = call "age364xa Configure Voltage Level.vi"("error in (no error)"=w425, "Level (0.0 Volts)"=0.0, "VISA session"=w419) -> ("error out"=w424:errorcluster, "dup VISA session"=w420:refnum<visa-resource-name>)  [unwired: 7 in]
        n324 = call "age364xa Configure Output Enabled.vi"("error in (no error)"=w424, "Output Enabled (F: Off)"=FALSE, "VISA session"=w420) -> ("error out"=w421:errorcluster, "dup VISA session"=w418:refnum<visa-resource-name>)  [unwired: 7 in]
      }
    }
    "Power OFF" <- w77
    "VDD Out Dup" <- w75
    n325 = Wait Until Next ms Multiple(millisecond multiple=u32 50) -> ()  [unwired: 1 out]
    "Status" <- "Idle....." ("Status")
  }
  n326 = VISA Write(VISA resource name=w20, write buffer="OUTP 0;", error in (no error)=w21) -> (VISA resource name out=w18:refnum<visa-resource-name>, error out=w22:errorcluster)  [unwired: 1 out]
  n327 = VISA Close(VISA resource name=w41, error in (no error)=w6) -> (error out=→"RFFE Out":errorcluster)
  n328 = VISA Close(VISA resource name=w25, error in (no error)=w6) -> (error out=→"2K Out":errorcluster)
  n329 = VISA Close(VISA resource name=w28, error in (no error)=w6) -> (error out=→"I2C Error Out":errorcluster)
  n330 = VISA Close(VISA resource name=w18, error in (no error)=w22) -> (error out=→"P/S Out":errorcluster)
